vi "FL30XX - Copy.VI"() -> ()   [LabVIEW 2015]
uses:
  board.vis/Globals.vi
panel:
  out "String":string="with int trig:\nset exp.time accordingly\ncheck with scope!"
  in  "BlockSyncStart":string(combo)="S1"
  out "TDC 2":u16
  out "TDC 1":u16
  in  "startevent":bool
  in  "Scan Trig Input Sel":string(combo)="I"
  in  "rep time":dbl=20.0 format="%.3f"
  in  "FFT mode":string(combo)="Full Binning"
  in  "shutter open":bool
  in  "value black":u32
  in  "value white":u32=65535
  in  "show greyscale viewer":bool
  out "mean 3":dbl=42.0 format="%0#.1f"
  out "tRMS 3":dbl=42.0 format="%0#.1f"
  out "meanB":dbl format="%0#.1f"
  out "tRMSB":dbl format="%0#.1f"
  in  "Pixel for Graph":u32(slide)=660 max=3000 scale=0.0..1087.0
  in  "fast test\ncontinuous":bool
  out "One Pixel Graph":u16[][](graph)=[[65535, 65535, 7490, 7490, 7489, 7487, 7484, 7472, 7491, 7479]]
  in  "refresh":bool
  out "C 8":bool
  out "C 7":bool
  out "C 6":bool
  out "C 5":bool=TRUE
  out "C 4":bool=TRUE
  out "C 3":bool
  out "C 2":bool
  out "(LastCAM) \n        C1":bool
  out "cool_temp Reg":u32=411900038 format="%032b"
  in  "cool":u8 caption="(0 to 7)"
  in  "Offset":bool
  out "Signal Cam 4":u16[](graph)
  out "Signal Cam 3":u16[](graph)
  out "mean 2":dbl=42.0 format="%0#.1f"
  out "meanA":dbl=nan format="%0#.1f"
  in  "TRMS Pix":u32=1060
  out "tRMS 2":dbl=42.0 format="%0#.1f"
  in  "Board select":string(combo)
  in  "Initialize":bool
  in  "pattern hex (2)":u16=100 format="%x"
  out "pattern dec 2":fxp<+,14,14>=100.0
  in  "ADC mode 2":enum32{"1", "2", "3"}(radio)=enum."3"
  in  "camera gain":bool
  in  "About S0":bool
  in  "send all":bool
  in  "DAC 8/ 1":u16=53010
  in  "DAC 3/ 1":u16=53045
  in  "DAC 7/ 1":u16=53015
  in  "DAC 2/ 1":u16=53185
  in  "DAC 6/ 1":u16=53110
  in  "DAC 1/ 1":u16=53100
  in  "DAC 5/ 1":u16=53005
  in  "DAC 4/ 1":u16=53190
  in  "custom patt: 14bits pattern hex (14bit)":u16=100 format="%x"
  out "pattern dec":fxp<+,14,14>
  in  "ADC mode":enum32{"1", "2", "3"}(radio)=enum."3"
  out "Signal Cam 2":u16[](graph)
  in  "ext. trig. slope":enum32{"1", "2", "3"}(radio)
  out "tRMSA":dbl format="%0#.1f"
  in  "is FFT":bool=TRUE
  in  "Gain":bool
  in  "framewise\ncontinuous":bool
  out "curr_read_block":u8
  out "Measure ON":bool
  in  "no.of blocks (nob)":u32=1
  in  "block":u32(slide)=1 max=10 scale=0.9..1.0
  out "Signal Board 2 / Cam1":u16[](graph)=[486, 486, 486, 486, 0, 0, 0, 52, 0, 692, 692, 490, 486, 482, 487, 490, 495, 482, 495, 487, 492, 486, 500, 497, 493, 487, 497, 490, 490, 489, 487, 489, 486, 486, 495, 492, 489, 490, 498, 492, 493, 490, 500, 487, 492, 486, 504, 489, 487, 487, 490, 487, 495, 490, 493, 493, 490, 490, 490, 492, 492, 490, 487, 486, 487, 482, 495, 487, 490, 484, 489, 481, 490, 484, 489, 484, 486, 490, 484, 487, 497, 484, 481, 479, 484, 481, 481, 492, 490, 484, 490, 490, 490, 481, 484, 482, 484, 484, 482, 482, 492, 482, 479, 481, 489, 481, 495, 484, 497, 482, 486, 484, 487, 486, 484, 484, 486, 479, 482, 473, 492, 486, 481, 486, 493, 481, 487, 474, 486, 487, 490, 473, 489, 486, 482, 486, 486, 486, 486, 479, 460, 478, 470, 484, 470, 478, 481, 481, 467, 481, 473, 484, 471, 479, 481, 473, 473, 473, 468, 467, 463, 473, 463, 473, 468, 473, 471, 478, 473, 476, 473, 473, 470, 474, 478, 474, 471, 470, 470, 467, 470, 486, 478, 468, 463, 473, 471, 481, 476, 476, 471, 473, 463, 473, 468, 478, 459, 463, 471, 482, 478, 484, 465, 476, 468, 470, 474, 478, 468, 468, 476, 478, 470, 471, 462, 467, 462, 470, 473, 471, 467, 476, 465, 463, 465, 470, 459, 471, 465, 462, 470, 471, 470, 478, 465, 474, 470, 471, 465, 474, 459, 468, 465, 474, 467, 468, 468, 467, 468, 460, 465, 479, 463, 470, 463, 460, 471, 478, 460, 468, 463, 467, 468, 474, 457, 457, 457, 538, 531, 544, 533, 558, 534, 557, 536, 547, 533, 547, 549, 544, 534, 544, 534, 542, 544, 544, 538, 541, 538, 547, 538, 542, 536, 545, 547, 552, 544, 542, 544, 542, 544, 544, 549, 549, 553, 550, 542, 550, 538, 545, 544, 541, 539, 545, 544, 539, 550, 544, 541, 549, 527, 542, 539, 541, 539, 539, 541, 542, 541, 544, 534, 538, 533, 534, 538, 544, 547, 541, 539, 547, 538, 538, 542, 542, 527, 536, 536, 544, 533, 533, 536, 541, 536, 542, 528, 541, 527, 534, 528, 541, 539, 549, 544, 550, 536, 542, 541, 550, 541, 538, 533, 539, 536, 530, 534, 539, 534, 542, 541, 547, 533, 538, 527, 539, 538, 541, 530, 542, 533, 534, 538, 536, 538, 538, 538, 530, 522, 531, 533, 544, 536, 536, 525, 536, 538, 536, 538, 533, 530, 538, 534, 536, 525, 533, 525, 530, 528, 531, 528, 527, 522, 528, 530, 523, 530, 541, 523, 527, 530, 536, 528, 536, 525, 530, 533, 542, 527, 536, 538, 531, 531, 523, 525, 538, 523, 533, 527, 538, 527, 528, 520, 533, 520, 536, 531, 534, 530, 534, 525, 525, 525, 522, 523, 536, 534, 527, 525, 525, 531, 538, 527, 528, 520, 523, 533, 534, 516, 523, 517, 525, 523, 527, 523, 528, 525, 520, 525, 523, 525, 533, 527, 533, 528, 527, 523, 530, 520, 530, 520, 527, 520, 527, 517, 525, 522, 527, 525, 534, 523, 523, 522, 517, 528, 534, 517, 522, 527, 523, 516, 527, 522, 522, 522, 615, 613, 620, 613, 626, 615, 628, 617, 624, 605, 621, 618, 617, 609, 618, 621, 617, 612, 613, 605, 612, 610, 626, 612, 621, 607, 620, 613, 613, 623, 629, 617, 617, 613, 626, 617, 621, 610, 617, 609, 621, 617, 618, 618, 613, 612, 618, 626, 623, 623, 623, 612, 620, 615, 623, 610, 620, 607, 615, 609, 613, 613, 617, 607, 617, 612, 610, 609, 617, 613, 613, 609, 617, 609, 612, 612, 618, 607, 615, 610, 615, 609, 620, 612, 612, 610, 618, 610, 609, 601, 601, 607, 613, 605, 613, 615, 615, 612, 609, 612, 615, 609, 601, 607, 612, 604, 612, 596, 613, 612, 610, 612, 617, 609, 609, 612, 612, 615, 613, 607, 610, 607, 609, 613, 610, 609, 609, 609, 602, 593, 605, 607, 609, 593, 609, 607, 610, 609, 610, 604, 594, 602, 610, 602, 607, 594, 613, 594, 604, 604, 607, 602, 594, 601, 609, 602, 601, 602, 609, 598, 605, 602, 605, 604, 609, 601, 604, 607, 615, 599, 607, 610, 609, 607, 610, 607, 610, 612, 605, 602, 610, 596, 602, 594, 607, 602, 605, 599, 610, 601, 607, 590, 594, 601, 594, 594, 604, 602, 596, 602, 605, 599, 594, 588, 604, 593, 598, 596, 601, 591, 601, 594, 601, 601, 599, 587, 598, 593, 594, 594, 599, 601, 598, 599, 598, 602, 605, 593, 602, 598, 601, 596, 609, 598, 593, 588, 596, 601, 601, 593, 601, 594, 598, 601, 599, 599, 604, 591, 596, 593, 601, 601, 612, 596, 596, 596, 598, 593, 596, 594, 591, 593, 602, 598, 602, 596, 601, 594, 590, 583, 593, 598, 593, 588, 602, 594, 585, 587, 602, 591, 593, 593, 593, 591, 585, 599, 601, 591, 593, 599, 598, 594, 593, 587, 596, 590, 591, 591, 604, 598, 594, 596, 599, 590, 602, 601, 590, 582, 599, 583, 593, 580, 598, 591, 590, 587, 593, 588, 587, 585, 594, 590, 583, 590, 594, 585, 588, 583, 593, 593, 588, 585, 590, 588, 590, 596, 599, 588, 588, 590, 591, 591, 585, 587, 596, 583, 590, 585, 585, 579, 583, 582, 588, 587, 590, 588, 591, 579, 583, 588, 590, 582, 587, 580, 587, 585, 587, 587, 598, 590, 585, 582, 587, 593, 590, 585, 588, 588, 587, 591, 587, 596, 596, 596, 650, 651, 661, 662, 658, 651, 656, 654, 656, 654, 658, 656, 650, 651, 650, 654, 650, 658, 661, 653, 659, 654, 656, 658, 651, 653, 656, 658, 654, 658, 654, 654, 658, 654, 662, 653, 656, 653, 656, 656, 667, 653, 658, 654, 645, 648, 658, 659, 656, 658, 653, 650, 658, 650, 651, 653, 661, 643, 653, 654, 658, 651, 658, 640, 661, 645, 640, 646, 648, 653, 648, 650, 656, 648, 648, 658, 658, 642, 648, 661, 658, 646, 650, 653, 650, 645, 643, 645, 653, 643, 642, 646, 654, 648, 646, 651, 656, 648, 656, 642, 648, 640, 648, 646, 654, 654, 640, 645, 654, 645, 654, 651, 651, 650, 651, 645, 642, 650, 653, 653, 648, 651, 656, 651, 650, 646, 646, 646, 481, 482, 478, 486, 486, 486, 486, 486, 486, 486, 486, 486, 486, 486, 486, 486, 486, 486, 486, 486, 486, 486, 486, 486, 486, 486, 486, 486, 486, 486, 486, 486, 486, 486, 486, 486, 486, 486, 486, 486, 486, 486, 486, 486, 486, 486, 486, 486, 486, 486, 486, 486, 486]
  out "Signal Board 1 / Cam1":u16[](graph)=[6280, 6289, 0, 1, 0, 10, 0, 0, 0, 0, 6308, 6311, 6305, 7303, 7306, 7305, 7298, 7309, 7318, 7312, 7317, 7306, 7300, 7301, 7287, 7279, 7286, 7287, 7288, 7284, 7286, 7285, 7270, 7282, 7282, 7261, 7269, 7267, 7263, 7261, 7274, 7261, 7263, 7266, 7264, 7271, 7253, 7245, 7254, 7250, 7257, 7250, 7235, 7242, 7238, 7242, 7236, 7239, 7237, 7237, 7237, 7238, 7231, 7224, 7231, 7221, 7222, 7224, 7210, 7213, 7215, 7217, 7219, 7225, 7215, 7211, 7219, 7221, 7209, 7207, 7208, 7206, 7194, 7206, 7213, 7200, 7196, 7193, 7205, 7190, 7191, 7203, 7205, 7199, 7187, 7196, 7198, 7179, 7188, 7191, 7186, 7185, 7189, 7184, 7181, 7177, 7192, 7182, 7181, 7173, 7180, 7174, 7171, 7173, 7169, 7174, 7166, 7161, 7138, 7168, 7165, 7168, 7167, 7171, 7157, 7169, 7155, 7156, 7173, 7153, 7166, 7156, 7153, 7150, 7155, 7150, 7153, 7142, 7138, 7135, 7140, 7156, 7152, 7147, 7145, 7142, 7147, 7135, 7133, 7146, 7135, 7152, 7134, 7129, 7141, 7137, 7140, 7130, 7139, 7144, 7129, 7142, 7133, 7131, 7121, 7130, 7125, 7135, 7139, 7126, 7131, 7134, 7138, 7127, 7120, 7137, 7121, 7133, 7144, 7136, 7135, 7133, 7138, 7134, 7135, 7141, 7145, 7149, 7150, 7144, 7143, 7157, 7165, 7156, 7152, 7146, 7152, 7150, 7155, 7159, 7150, 7160, 7145, 7139, 7147, 7154, 7134, 7153, 7144, 7138, 7141, 7146, 7148, 7134, 7148, 7140, 7153, 7138, 7143, 7134, 7155, 7157, 7153, 7147, 7149, 7150, 7151, 7141, 7135, 7142, 7136, 7146, 7143, 7152, 7147, 7139, 7144, 7152, 7150, 7129, 7136, 7137, 7149, 7145, 7132, 7144, 7138, 7141, 7145, 7142, 7141, 7145, 7142, 7140, 7143, 7138, 7145, 7154, 7139, 7148, 7149, 7150, 7135, 7149, 7145, 7151, 7151, 7147, 7143, 7148, 7145, 7142, 7144, 7149, 7158, 7148, 7149, 7148, 7151, 7154, 7148, 7139, 7144, 7142, 7145, 7142, 7150, 7154, 7138, 7142, 7152, 7145, 7146, 7147, 7146, 7140, 7144, 7146, 7148, 7152, 7152, 7159, 7154, 7146, 7155, 7157, 7147, 7153, 7146, 7156, 7155, 7153, 7148, 7153, 7154, 7159, 7155, 7154, 7157, 7152, 7157, 7155, 7147, 7154, 7154, 7151, 7154, 7168, 7167, 7164, 7168, 7161, 7165, 7168, 7147, 7156, 7157, 7162, 7160, 7160, 7164, 7169, 7163, 7168, 7170, 7161, 7174, 7162, 7159, 7166, 7167, 7162, 7169, 7168, 7158, 7162, 7163, 7174, 7160, 7158, 7167, 7168, 7176, 7178, 7162, 7176, 7176, 7158, 7178, 7166, 7174, 7162, 7168, 7186, 7170, 7171, 7163, 7176, 7158, 7177, 7178, 7169, 7166, 7168, 7165, 7179, 7174, 7177, 7180, 7186, 7190, 7181, 7180, 7181, 7169, 7179, 7174, 7178, 7196, 7183, 7189, 7193, 7187, 7194, 7184, 7185, 7184, 7196, 7198, 7193, 7202, 7198, 7203, 7197, 7187, 7200, 7197, 7197, 7205, 7201, 7206, 7212, 7186, 7199, 7206, 7196, 7212, 7213, 7217, 7209, 7221, 7204, 7212, 7209, 7218, 7220, 7215, 7222, 7228, 7218, 7223, 7218, 7231, 7219, 7227, 7219, 7223, 7228, 7231, 7224, 7234, 7236, 7240, 7227, 7237, 7243, 7241, 7240, 7228, 7238, 7233, 7241, 7233, 7238, 7244, 7240, 7240, 7232, 7252, 7238, 7247, 7249, 7249, 7247, 7248, 7259, 7250, 7256, 7256, 7263, 7258, 7259, 7261, 7266, 7274, 7271, 7262, 7261, 7258, 7259, 7266, 7269, 7274, 7271, 7280, 7282, 7271, 7290, 7275, 7288, 7288, 7287, 7286, 7275, 7297, 7289, 7286, 7289, 7297, 7284, 7307, 7299, 7295, 7293, 7311, 7298, 7297, 7305, 7310, 7298, 7306, 7306, 7320, 7310, 7313, 7320, 7313, 7312, 7313, 7313, 7325, 7321, 7325, 7309, 7328, 7335, 7326, 7321, 7339, 7324, 7332, 7333, 7333, 7334, 7343, 7331, 7364, 7337, 7328, 7338, 7348, 7355, 7341, 7350, 7368, 7369, 7362, 7361, 7369, 7368, 7357, 7377, 7362, 7365, 7364, 7371, 7363, 7371, 7384, 7374, 7385, 7370, 7370, 7387, 7394, 7380, 7383, 7398, 7395, 7393, 7389, 7402, 7402, 7394, 7387, 7406, 7388, 7403, 7403, 7404, 7404, 7413, 7401, 7407, 7410, 7406, 7405, 7402, 7408, 7409, 7415, 7420, 7416, 7416, 7419, 7422, 7408, 7426, 7424, 7428, 7431, 7420, 7433, 7430, 7421, 7427, 7438, 7431, 7440, 7433, 7440, 7442, 7446, 7441, 7453, 7443, 7441, 7450, 7447, 7459, 7441, 7457, 7461, 7447, 7448, 7461, 7455, 7467, 7465, 7450, 7466, 7463, 7464, 7463, 7461, 7466, 7465, 7478, 7479, 7466, 7471, 7482, 7497, 7463, 7484, 7490, 7495, 7474, 7488, 7489, 7479, 7498, 7493, 7489, 7490, 7498, 7487, 7487, 7495, 7501, 7491, 7491, 7509, 7496, 7507, 7506, 7495, 7500, 7505, 7505, 7500, 7511, 7513, 7504, 7504, 7509, 7520, 7526, 7518, 7517, 7521, 7519, 7514, 7534, 7523, 7518, 7521, 7529, 7536, 7530, 7534, 7532, 7510, 7521, 7529, 7530, 7534, 7522, 7545, 7530, 7531, 7539, 7540, 7553, 7545, 7542, 7531, 7542, 7540, 7552, 7565, 7548, 7554, 7551, 7554, 7548, 7564, 7574, 7565, 7555, 7560, 7572, 7561, 7563, 7571, 7556, 7569, 7571, 7568, 7569, 7585, 7572, 7577, 7574, 7568, 7591, 7583, 7579, 7580, 7590, 7586, 7592, 7604, 7604, 7597, 7593, 7600, 7606, 7620, 7616, 7618, 7602, 7616, 7621, 7609, 7633, 7618, 7629, 7640, 7638, 7630, 7634, 7630, 7631, 7642, 7639, 7627, 7635, 7646, 7656, 7663, 7653, 7654, 7645, 7655, 7656, 7653, 7665, 7659, 7654, 7671, 7661, 7672, 7683, 7675, 7677, 7666, 7669, 7654, 7678, 7676, 7674, 7678, 7679, 7674, 7672, 7677, 7693, 7688, 7685, 7681, 7691, 7693, 7702, 7691, 7691, 7698, 7694, 7696, 7698, 7682, 7694, 7698, 7689, 7699, 7699, 7682, 7700, 7689, 7696, 7705, 7686, 7702, 7693, 7686, 7689, 7687, 7685, 7694, 7705, 7689, 7694, 7692, 7680, 7706, 7694, 7690, 7691, 7683, 7686, 7676, 7662, 7664, 7676, 7655, 7674, 7650, 7660, 7644, 7643, 7642, 7635, 7625, 7632, 7621, 7605, 7603, 7597, 7598, 7582, 7575, 7568, 7568, 7568, 7565, 7554, 7533, 7529, 7532, 7507, 7510, 7508, 7509, 7491, 7470, 7468, 7464, 7465, 7445, 7433, 7425, 7409, 7410, 7398, 7399, 7379, 7373, 7365, 7346, 7341, 7322, 7325, 7308, 7296, 7289, 7281, 7271, 7251, 7253, 7243, 7223, 7201, 7189, 7167, 7174, 7161, 7135, 7122, 7095, 7082, 7070, 7055, 7045, 7017, 6997, 6995, 6973, 6966, 6960, 6928, 6942, 6926, 6922, 6915, 6901, 6896, 6883, 6873, 6879, 6874, 6860, 6851, 6855, 6841, 6833, 6827, 6822, 6813, 6811, 6800, 6810, 6803, 6788, 6782, 6786, 6772, 6767, 6771, 6765, 6752, 6758, 6753, 6743, 6737, 6745, 6733, 6725, 6717, 6728, 6717, 6720, 6711, 6708, 6706, 6702, 6705, 6695, 6687, 6687, 6689, 6676, 6676, 6679, 6665, 6663, 6640, 6654, 6656, 6650, 6644, 6645, 6644, 6639, 6631, 6634, 6631, 6620, 6626, 6621, 6620, 6611, 6612, 6609, 6615, 6607, 6605, 6596, 6604, 6596, 6589, 6586, 6585, 6589, 6583, 6582, 6576, 6578, 6563, 6579, 6574, 6565, 6565, 6562, 6560, 6559, 6551, 6547, 6556, 6546, 6549, 6535, 6533, 6539, 6541, 6540, 6527, 6525, 6528, 6523, 6525, 6524, 6520, 6522, 6519, 6518, 6505, 6510, 6503, 6502, 6286, 6279, 6278, 6281, 6279, 6279, 6286, 6279, 6280, 6282, 6285, 6282, 6284, 6285, 6282, 6280, 6285, 6281, 6283, 6283, 6280, 6276, 6282, 6282, 6283, 6276, 6281, 6277, 6282, 6277, 6279, 6277, 6281, 0, 0, 65535, 65535, 6279, 6283]
  out "# boards \ndetected":u8=1
  in  "alloc mem":bool
  out "FREE \nRAM MB":dbl=29529.31640625
  out "BUILT-IN\nRAM MB":dbl=32640.29296875
  out "SEC":dbl=0.005
  out "MB RAM":dbl=0.0103759765625
  in  "DAT in 10ns":u32
  in  "stop all":bool
  in  "start":bool
  in  "sample":u32(slide)=10 max=3000 scale=0.9..4.0
  in  "no.of samples (nos)":u32=4
  in  "exposuretime[ms]":dbl=1.0 format="%.3f"
  # "Put the right values in this frame\n           and press \"Initialize\""
  # "press Esc to\nstop measurement"
  # "exit here"
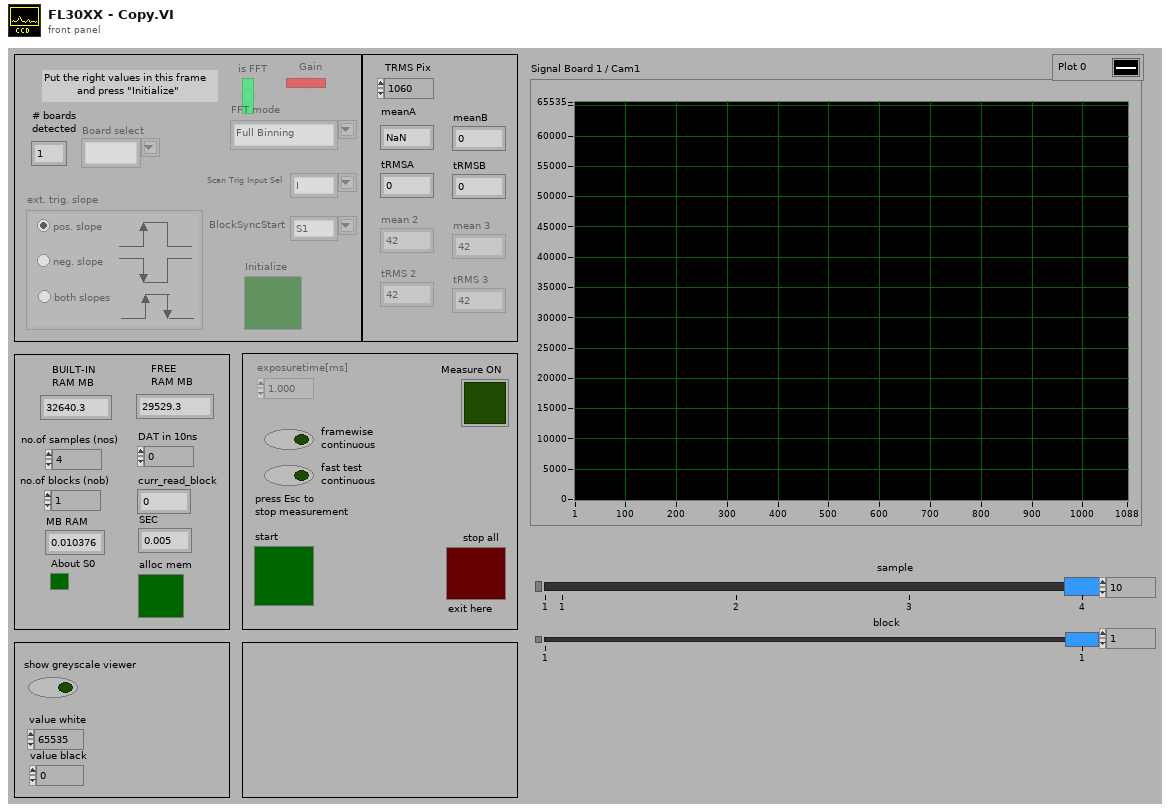
[diagram p1: front panel]
types:
  T1 = enum8{"Enabled", "Disabled", "Disabled and Grayed Out"}
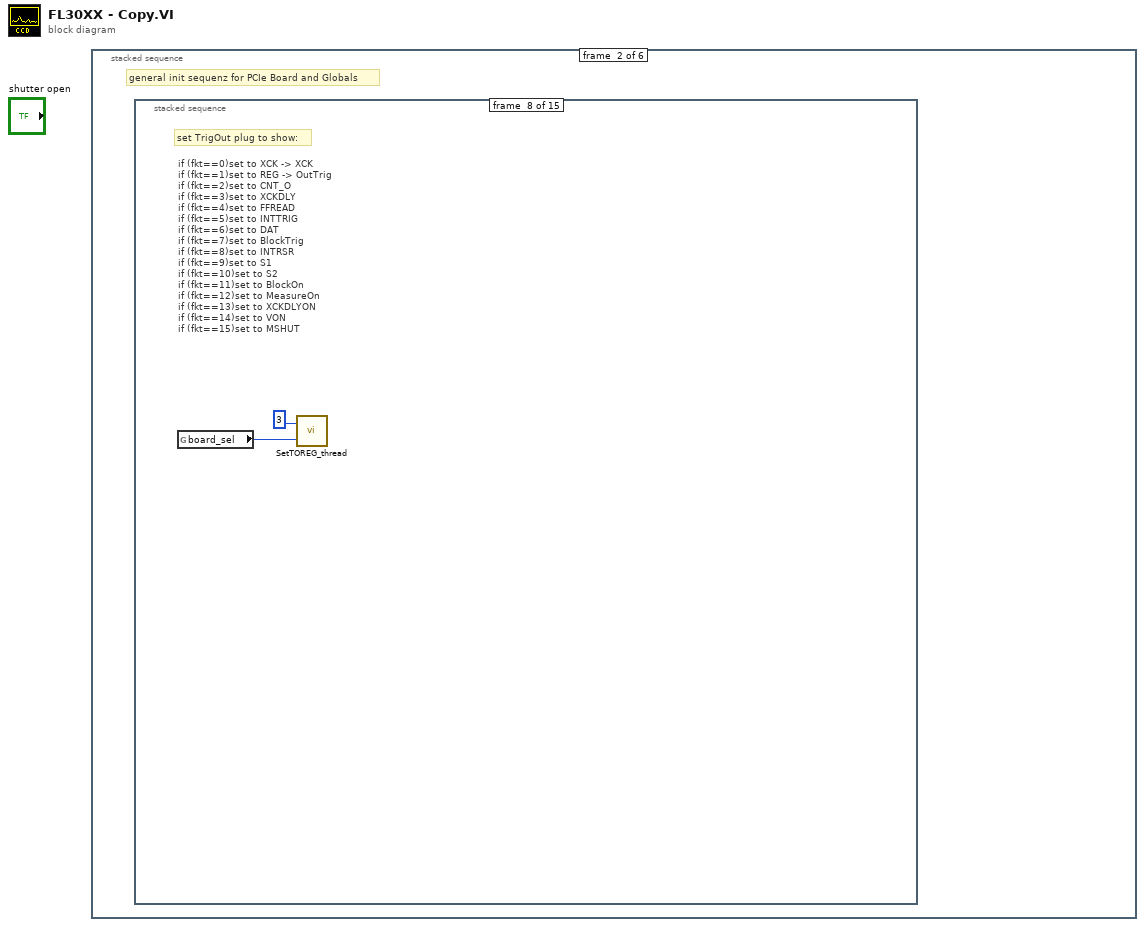
[diagram p0: block diagram]
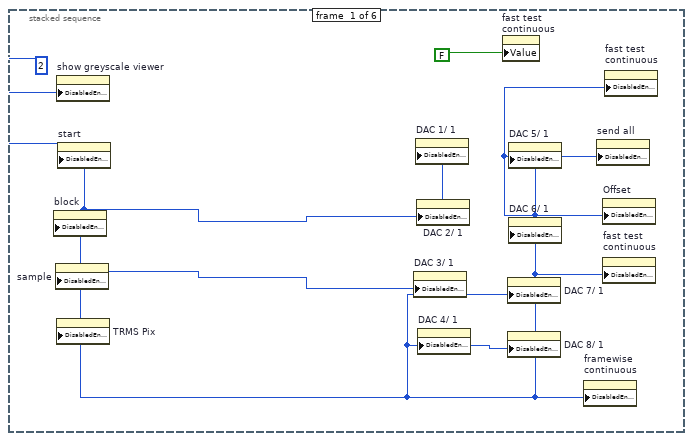
[diagram p2: hidden frame]
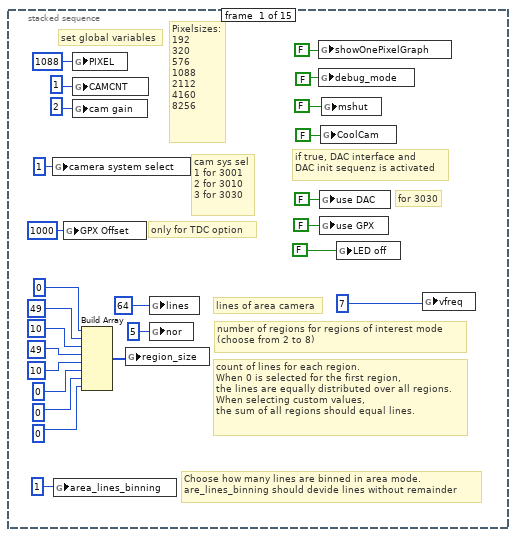
[diagram p3: hidden frame]
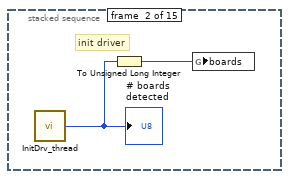
[diagram p4: hidden frame]
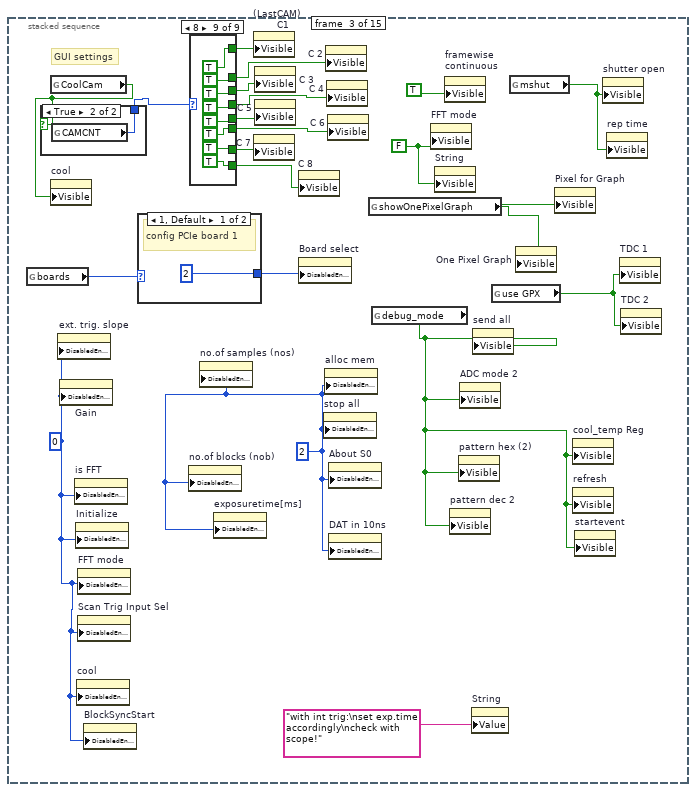
[diagram p5: hidden frame]
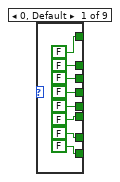
[diagram p6: hidden frame]
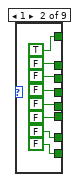
[diagram p7: hidden frame]
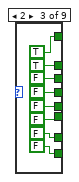
[diagram p8: hidden frame]
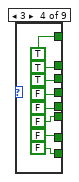
[diagram p9: hidden frame]
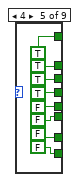
[diagram p10: hidden frame]
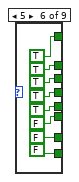
[diagram p11: hidden frame]
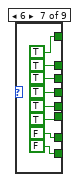
[diagram p12: hidden frame]
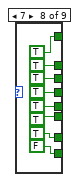
[diagram p13: hidden frame]
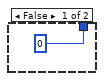
[diagram p14: hidden frame]
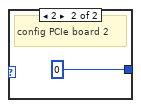
[diagram p15: hidden frame]
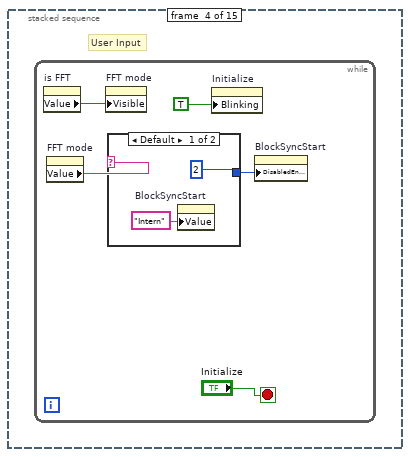
[diagram p16: hidden frame]
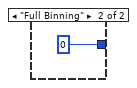
[diagram p17: hidden frame]
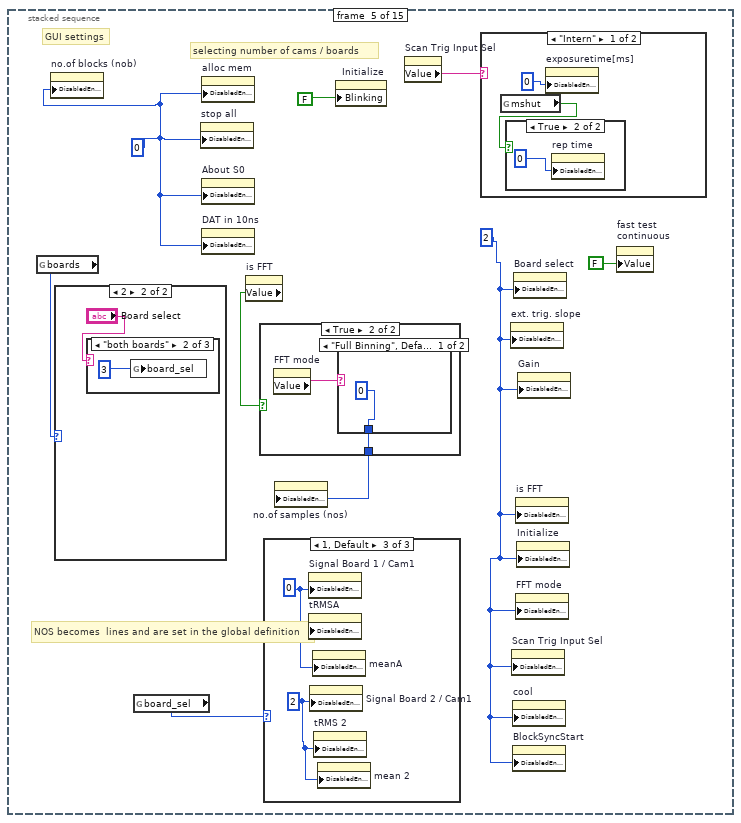
[diagram p18: hidden frame]
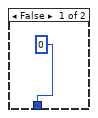
[diagram p19: hidden frame]
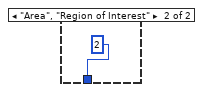
[diagram p20: hidden frame]
diagram:
  n1 = stacked-sequence {
    frame #0 {
      w1 = 2
      n2 = property on="block" class="Slide (strict)"("DisabledEnum"=w1) -> ()  [unwired: 2 in, 2 out]
      n3 = property on="sample" class="Slide (strict)"("DisabledEnum"=w1) -> ()  [unwired: 2 in, 2 out]
      n4 = property on="show greyscale viewer" class="Bool (strict)"("DisabledEnum"=w1) -> ()  [unwired: 2 in, 2 out]
      n5 = property on="TRMS Pix" class="DigNum (strict)"("DisabledEnum"=w1) -> ()  [unwired: 2 in, 2 out]
      n6 = property on="start" class="Bool (strict)"("DisabledEnum"=w1) -> ()  [unwired: 2 in, 2 out]
      n7 = property on="DAC 3/ 1" class="DigNum (strict)"("DisabledEnum"=w1) -> ()  [unwired: 2 in, 2 out]
      n8 = property on="DAC 1/ 1" class="DigNum (strict)"("DisabledEnum"=w1) -> ()  [unwired: 2 in, 2 out]
      n9 = property on="DAC 2/ 1" class="DigNum (strict)"("DisabledEnum"=w1) -> ()  [unwired: 2 in, 2 out]
      n10 = property on="DAC 4/ 1" class="DigNum (strict)"("DisabledEnum"=w1) -> ()  [unwired: 2 in, 2 out]
      n11 = property on="fast test\ncontinuous" class="Bool (strict)"("Value"=FALSE) -> ()  [unwired: 2 in, 2 out]
      n12 = property on="DAC 7/ 1" class="DigNum (strict)"("DisabledEnum"=w1) -> ()  [unwired: 2 in, 2 out]
      n13 = property on="DAC 8/ 1" class="DigNum (strict)"("DisabledEnum"=w1) -> ()  [unwired: 2 in, 2 out]
      n14 = property on="DAC 5/ 1" class="DigNum (strict)"("DisabledEnum"=w1) -> ()  [unwired: 2 in, 2 out]
      n15 = property on="DAC 6/ 1" class="DigNum (strict)"("DisabledEnum"=w1) -> ()  [unwired: 2 in, 2 out]
      n16 = property on="framewise\ncontinuous" class="Bool (strict)"("DisabledEnum"=w1) -> ()  [unwired: 2 in, 2 out]
      n17 = property on="send all" class="Bool (strict)"("DisabledEnum"=w1) -> ()  [unwired: 2 in, 2 out]
      n18 = property on="Offset" class="Bool (strict)"("DisabledEnum"=w1) -> ()  [unwired: 2 in, 2 out]
      n19 = property on="fast test\ncontinuous" class="Bool (strict)"("DisabledEnum"=w1) -> ()  [unwired: 2 in, 2 out]
      n20 = property on="fast test\ncontinuous" class="Bool (strict)"("DisabledEnum"=w1) -> ()  [unwired: 2 in, 2 out]
    }
    frame #1 {
      # "general init sequenz for PCIe Board and Globals"
      n21 = stacked-sequence {
        frame #0 {
          # "Choose how many lines are binned in area mode.\nare_lines_binning should devide lines without remainder"
          # "count of lines for each region.\nWhen 0 is selected for the first region,\nthe lines are equally distributed over all regions.\nWhen selecting custom values,\nthe sum of all regions should equal lines."
          # "number of regions for regions of interest mode\n(choose from 2 to 8)"
          # "lines of area camera"
          # "only for TDC option"
          # "Pixelsizes:\n192\n320\n576\n1088\n2112\n4160\n8256"
          # "if true, DAC interface and \nDAC init sequenz is activated"
          # "for 3030"
          # "set global variables"
          # "cam sys sel\n1 for 3001\n2 for 3010\n3 for 3030"
          n22 = global write "Globals.vi" "camera system select"(u8 1) -> ()
          n23 = global write "Globals.vi" "area_lines_binning"(u32 1) -> ()
          n24 = global write "Globals.vi" "GPX Offset"(u32 1000) -> ()
          n25 = global write "Globals.vi" "PIXEL"(u32 1088) -> ()
          n26 = global write "Globals.vi" "CAMCNT"(u32 1) -> ()
          n27 = global write "Globals.vi" "cam gain"(u32 2) -> ()
          n28 = Build Array(u8 0, u8 49, u8 10, u8 49, u8 10, u8 0, u8 0, u8 0) -> (w6:u8[])
          n29 = global write "Globals.vi" "region_size"(w6) -> ()
          n30 = global write "Globals.vi" "lines"(u32 64) -> ()
          n31 = global write "Globals.vi" "nor"(u32 5) -> ()
          n32 = global write "Globals.vi" "showOnePixelGraph"(FALSE) -> ()
          n33 = global write "Globals.vi" "debug_mode"(FALSE) -> ()
          n34 = global write "Globals.vi" "use DAC"(FALSE) -> ()
          n35 = global write "Globals.vi" "use GPX"(FALSE) -> ()
          n36 = global write "Globals.vi" "CoolCam"(FALSE) -> ()
          n37 = global write "Globals.vi" "mshut"(FALSE) -> ()
          n38 = global write "Globals.vi" "LED off"(FALSE) -> ()
          n39 = global write "Globals.vi" "vfreq"(u8 7) -> ()
        }
        frame #1 {
          # "init driver"
          n40 = call "InitDrv_thread.vi"() -> ("Boards"=w28:u8)  [unwired: 1 in]
          "# boards \ndetected" <- w28
          n41 = To Unsigned Long Integer(number=w28) -> (unsigned 32bit integer=w29:u32)
          n42 = global write "Globals.vi" "boards"(w29) -> ()
        }
        frame #2 {
          w32 = FALSE
          w30 = 0
          w33 = 2
          # "GUI settings"
          n43 = global read "Globals.vi" "boards"() -> (w49:u32)
          n44 = global read "Globals.vi" "CoolCam"() -> (w38:bool)
          n45 = case shown="True" w38 {
            tunnel: [u32 0 w124] -> w47
            frame False {
            }
            frame True {
              n46 = global read "Globals.vi" "CAMCNT"() -> (w124:u32)
            }
          }
          n47 = property on="cool" class="DigNum (strict)"("Visible"=w38) -> ()  [unwired: 2 in, 2 out]
          n48 = property on="ext. trig. slope" class="RadioBtnsControl (strict)"("DisabledEnum"=w30) -> ()  [unwired: 2 in, 2 out]
          n49 = property on="Gain" class="Bool (strict)"("DisabledEnum"=w30) -> ()  [unwired: 2 in, 2 out]
          n50 = property on="is FFT" class="Bool (strict)"("DisabledEnum"=w30) -> ()  [unwired: 2 in, 2 out]
          n51 = property on="Initialize" class="Bool (strict)"("DisabledEnum"=w30) -> ()  [unwired: 2 in, 2 out]
          n52 = property on="cool" class="DigNum (strict)"("DisabledEnum"=w30) -> ()  [unwired: 2 in, 2 out]
          n53 = property on="FFT mode" class="CmbBox"("DisabledEnum"=w30) -> ()  [unwired: 2 in, 2 out]
          n54 = property on="Scan Trig Input Sel" class="CmbBox"("DisabledEnum"=w30) -> ()  [unwired: 2 in, 2 out]
          n55 = property on="BlockSyncStart" class="CmbBox"("DisabledEnum"=w30) -> ()  [unwired: 2 in, 2 out]
          n56 = case shown="1, Default" w49 {
            tunnel: [2 0] -> w50
            frame 1, Default {
              # "config PCIe board 1"
            }
            frame 2 {
              # "config PCIe board 2"
            }
          }
          n57 = property on="no.of blocks (nob)" class="DigNum (strict)"("DisabledEnum"=w33) -> ()  [unwired: 2 in, 2 out]
          n58 = case shown="8" w47 {
            tunnel: [FALSE TRUE TRUE TRUE TRUE TRUE TRUE TRUE TRUE] -> w46
            tunnel: [FALSE FALSE FALSE TRUE TRUE TRUE TRUE TRUE TRUE] -> w45
            tunnel: [FALSE FALSE FALSE FALSE TRUE TRUE TRUE TRUE TRUE] -> w44
            tunnel: [FALSE FALSE FALSE FALSE FALSE TRUE TRUE TRUE TRUE] -> w43
            tunnel: [FALSE FALSE FALSE FALSE FALSE FALSE TRUE TRUE TRUE] -> w42
            tunnel: [FALSE FALSE FALSE FALSE FALSE FALSE FALSE TRUE TRUE] -> w41
            tunnel: [FALSE FALSE FALSE FALSE FALSE FALSE FALSE FALSE TRUE] -> w40
            tunnel: [FALSE FALSE TRUE TRUE TRUE TRUE TRUE TRUE TRUE] -> w39
            frame 0, Default {
            }
            frame 1 {
            }
            frame 2 {
            }
            frame 3 {
            }
            frame 4 {
            }
            frame 5 {
            }
            frame 6 {
            }
            frame 7 {
            }
            frame 8 {
            }
          }
          n59 = property on="no.of samples (nos)" class="DigNum (strict)"("DisabledEnum"=w33) -> ()  [unwired: 2 in, 2 out]
          n60 = property on="exposuretime[ms]" class="DigNum (strict)"("DisabledEnum"=w33) -> ()  [unwired: 2 in, 2 out]
          n61 = property on="(LastCAM) \n        C1" class="Bool (strict)"("Visible"=w46) -> ()  [unwired: 2 in, 2 out]
          n62 = property on="C 7" class="Bool (strict)"("Visible"=w41) -> ()  [unwired: 2 in, 2 out]
          n63 = property on="C 3" class="Bool (strict)"("Visible"=w45) -> ()  [unwired: 2 in, 2 out]
          n64 = property on="C 5" class="Bool (strict)"("Visible"=w43) -> ()  [unwired: 2 in, 2 out]
          n65 = property on="C 8" class="Bool (strict)"("Visible"=w40) -> ()  [unwired: 2 in, 2 out]
          n66 = property on="Board select" class="CmbBox"("DisabledEnum"=w50) -> ()  [unwired: 2 in, 2 out]
          n67 = property on="stop all" class="Bool (strict)"("DisabledEnum"=w33) -> ()  [unwired: 2 in, 2 out]
          n68 = property on="alloc mem" class="Bool (strict)"("DisabledEnum"=w33) -> ()  [unwired: 2 in, 2 out]
          n69 = property on="C 2" class="Bool (strict)"("Visible"=w39) -> ()  [unwired: 2 in, 2 out]
          n70 = property on="C 4" class="Bool (strict)"("Visible"=w44) -> ()  [unwired: 2 in, 2 out]
          n71 = property on="C 6" class="Bool (strict)"("Visible"=w42) -> ()  [unwired: 2 in, 2 out]
          n72 = property on="About S0" class="Bool (strict)"("DisabledEnum"=w33) -> ()  [unwired: 2 in, 2 out]
          n73 = property on="DAT in 10ns" class="DigNum (strict)"("DisabledEnum"=w33) -> ()  [unwired: 2 in, 2 out]
          n74 = global read "Globals.vi" "showOnePixelGraph"() -> (w37:bool)
          n75 = global read "Globals.vi" "debug_mode"() -> (w35:bool)
          n76 = property on="FFT mode" class="CmbBox"("Visible"=w32) -> ()  [unwired: 2 in, 2 out]
          n77 = property on="String" class="Str"("Visible"=w32) -> ()  [unwired: 2 in, 2 out]
          n78 = property on="framewise\ncontinuous" class="Bool (strict)"("Visible"=TRUE) -> ()  [unwired: 2 in, 2 out]
          n79 = property on="pattern dec 2" class="DigNum (strict)"("Visible"=w35) -> ()  [unwired: 2 in, 2 out]
          n80 = property on="pattern hex (2)" class="DigNum (strict)"("Visible"=w35) -> ()  [unwired: 2 in, 2 out]
          n81 = property on="ADC mode 2" class="RadioBtnsControl (strict)"("Visible"=w35) -> ()  [unwired: 2 in, 2 out]
          n82 = property on="String" class="Str"("Value"="with int trig:\nset exp.time accordingly\ncheck with scope!") -> ()  [unwired: 2 in, 2 out]
          n83 = property on="send all" class="Bool (strict)"("Visible"=w35) -> ()  [unwired: 2 in, 2 out]
          n84 = global read "Globals.vi" "use GPX"() -> (w34:bool)
          n85 = global read "Globals.vi" "mshut"() -> (w36:bool)
          n86 = property on="One Pixel Graph" class="WFGraph (strict)"("Visible"=w37) -> ()  [unwired: 2 in, 2 out]
          n87 = property on="Pixel for Graph" class="Slide (strict)"("Visible"=w37) -> ()  [unwired: 2 in, 2 out]
          n88 = property on="cool_temp Reg" class="DigNum (strict)"("Visible"=w35) -> ()  [unwired: 2 in, 2 out]
          n89 = property on="refresh" class="Bool (strict)"("Visible"=w35) -> ()  [unwired: 2 in, 2 out]
          n90 = property on="startevent" class="Bool (strict)"("Visible"=w35) -> ()  [unwired: 2 in, 2 out]
          n91 = property on="shutter open" class="Bool (strict)"("Visible"=w36) -> ()  [unwired: 2 in, 2 out]
          n92 = property on="rep time" class="DigNum (strict)"("Visible"=w36) -> ()  [unwired: 2 in, 2 out]
          n93 = property on="TDC 1" class="DigNum (strict)"("Visible"=w34) -> ()  [unwired: 2 in, 2 out]
          n94 = property on="TDC 2" class="DigNum (strict)"("Visible"=w34) -> ()  [unwired: 2 in, 2 out]
        }
        frame #3 {
          # "User Input"
          n95 = while {
            stop <- "Initialize" stop-if-true
            n96 = property on="is FFT" class="Bool (strict)"() -> ("Value"=w129:bool)  [unwired: 2 in, 2 out]
            n97 = property on="FFT mode" class="CmbBox"() -> ("Value"=w128:string)  [unwired: 2 in, 2 out]
            n98 = property on="FFT mode" class="CmbBox"("Visible"=w129) -> ()  [unwired: 2 in, 2 out]
            n99 = case shown="Default" w128 {
              tunnel: [2 0] -> w127
              frame Default {
                n100 = property on="BlockSyncStart" class="CmbBox"("Value"="Intern") -> ()  [unwired: 2 in, 2 out]
              }
              frame "Full Binning" {
              }
            }
            n101 = property on="Initialize" class="Bool (strict)"("Blinking"=TRUE) -> ()  [unwired: 2 in, 2 out]
            n102 = property on="BlockSyncStart" class="CmbBox"("DisabledEnum"=w127) -> ()  [unwired: 2 in, 2 out]
          }
        }
        frame #4 {
          w136 = u8 2
          w143 = i8 0
          # "NOS becomes  lines and are set in the global definition"
          # "GUI settings"
          # "selecting number of cams / boards"
          n103 = global read "Globals.vi" "boards"() -> (w141:u32)
          n104 = property on="no.of blocks (nob)" class="DigNum (strict)"("DisabledEnum"=w143) -> ()  [unwired: 2 in, 2 out]
          n105 = case shown="2" w141 {
            frame 1, Default {
              n106 = global write "Globals.vi" "board_sel"(u32 1) -> ()
            }
            frame 2 {
              n107 = case shown="\"both boards\"" "Board select" {
                frame "board 2" {
                  n108 = global write "Globals.vi" "board_sel"(u32 2) -> ()
                }
                frame "both boards" {
                  n109 = global write "Globals.vi" "board_sel"(u32 3) -> ()
                }
                frame "board 1", Default {
                  n110 = global write "Globals.vi" "board_sel"(u32 1) -> ()
                }
              }
            }
          }
          n111 = global read "Globals.vi" "board_sel"() -> (w140:u32)
          n112 = property on="stop all" class="Bool (strict)"("DisabledEnum"=w143) -> ()  [unwired: 2 in, 2 out]
          n113 = property on="alloc mem" class="Bool (strict)"("DisabledEnum"=w143) -> ()  [unwired: 2 in, 2 out]
          n114 = property on="About S0" class="Bool (strict)"("DisabledEnum"=w143) -> ()  [unwired: 2 in, 2 out]
          n115 = property on="DAT in 10ns" class="DigNum (strict)"("DisabledEnum"=w143) -> ()  [unwired: 2 in, 2 out]
          n116 = property on="is FFT" class="Bool (strict)"() -> ("Value"=w137:bool)  [unwired: 2 in, 2 out]
          n117 = case shown="True" w137 {
            tunnel: [u8 0 w145] -> w138
            frame False {
            }
            frame True {
              n118 = property on="FFT mode" class="CmbBox"() -> ("Value"=w146:string)  [unwired: 2 in, 2 out]
              n119 = case shown="\"Full Binning\", Default" w146 {
                tunnel: [i8 0 i8 2] -> w145
                frame "Full Binning", Default {
                }
                frame "Area", "Region of Interest" {
                }
              }
            }
          }
          n120 = case shown="1, Default" w140 {
            frame 2 {
              w157 = 0
              w158 = 2
              n121 = property on="Signal Board 1 / Cam1" class="WFGraph (strict)"("DisabledEnum"=w158) -> ()  [unwired: 2 in, 2 out]
              n122 = property on="tRMSA" class="DigNum (strict)"("DisabledEnum"=w158) -> ()  [unwired: 2 in, 2 out]
              n123 = property on="Signal Board 2 / Cam1" class="WFGraph (strict)"("DisabledEnum"=w157) -> ()  [unwired: 2 in, 2 out]
              n124 = property on="meanA" class="DigNum (strict)"("DisabledEnum"=w158) -> ()  [unwired: 2 in, 2 out]
              n125 = property on="tRMS 2" class="DigNum (strict)"("DisabledEnum"=w157) -> ()  [unwired: 2 in, 2 out]
              n126 = property on="mean 2" class="DigNum (strict)"("DisabledEnum"=w157) -> ()  [unwired: 2 in, 2 out]
            }
            frame 3 {
              w159 = 0
              w160 = 0
              n127 = property on="Signal Board 1 / Cam1" class="WFGraph (strict)"("DisabledEnum"=w160) -> ()  [unwired: 2 in, 2 out]
              n128 = property on="tRMSA" class="DigNum (strict)"("DisabledEnum"=w160) -> ()  [unwired: 2 in, 2 out]
              n129 = property on="Signal Board 2 / Cam1" class="WFGraph (strict)"("DisabledEnum"=w159) -> ()  [unwired: 2 in, 2 out]
              n130 = property on="meanA" class="DigNum (strict)"("DisabledEnum"=w160) -> ()  [unwired: 2 in, 2 out]
              n131 = property on="tRMS 2" class="DigNum (strict)"("DisabledEnum"=w159) -> ()  [unwired: 2 in, 2 out]
              n132 = property on="mean 2" class="DigNum (strict)"("DisabledEnum"=w159) -> ()  [unwired: 2 in, 2 out]
            }
            frame 1, Default {
              w161 = 2
              w162 = 0
              n133 = property on="Signal Board 1 / Cam1" class="WFGraph (strict)"("DisabledEnum"=w162) -> ()  [unwired: 2 in, 2 out]
              n134 = property on="tRMSA" class="DigNum (strict)"("DisabledEnum"=w162) -> ()  [unwired: 2 in, 2 out]
              n135 = property on="Signal Board 2 / Cam1" class="WFGraph (strict)"("DisabledEnum"=w161) -> ()  [unwired: 2 in, 2 out]
              n136 = property on="meanA" class="DigNum (strict)"("DisabledEnum"=w162) -> ()  [unwired: 2 in, 2 out]
              n137 = property on="tRMS 2" class="DigNum (strict)"("DisabledEnum"=w161) -> ()  [unwired: 2 in, 2 out]
              n138 = property on="mean 2" class="DigNum (strict)"("DisabledEnum"=w161) -> ()  [unwired: 2 in, 2 out]
            }
          }
          n139 = property on="no.of samples (nos)" class="DigNum (strict)"("DisabledEnum"=w138) -> ()  [unwired: 2 in, 2 out]
          n140 = property on="Initialize" class="Bool (strict)"("Blinking"=FALSE) -> ()  [unwired: 2 in, 2 out]
          n141 = property on="Scan Trig Input Sel" class="CmbBox"() -> ("Value"=w135:string)  [unwired: 2 in, 2 out]
          n142 = case shown="\"Intern\"" w135 {
            frame "Intern" {
              n143 = global read "Globals.vi" "mshut"() -> (w149:bool)
              n144 = case shown="True" w149 {
                frame False {
                  n145 = property on="rep time" class="DigNum (strict)"("DisabledEnum"=i8 2) -> ()  [unwired: 2 in, 2 out]
                }
                frame True {
                  n146 = property on="rep time" class="DigNum (strict)"("DisabledEnum"=i8 0) -> ()  [unwired: 2 in, 2 out]
                }
              }
              n147 = property on="exposuretime[ms]" class="DigNum (strict)"("DisabledEnum"=i8 0) -> ()  [unwired: 2 in, 2 out]
            }
            frame Default {
              n148 = global read "Globals.vi" "mshut"() -> (w153:bool)
              n149 = case shown="False" w153 {
                frame False {
                  n150 = property on="exposuretime[ms]" class="DigNum (strict)"("DisabledEnum"=i8 2) -> ()  [unwired: 2 in, 2 out]
                }
                frame True {
                  n151 = property on="exposuretime[ms]" class="DigNum (strict)"("DisabledEnum"=i8 0) -> ()  [unwired: 2 in, 2 out]
                }
              }
              n152 = property on="rep time" class="DigNum (strict)"("DisabledEnum"=i8 2) -> ()  [unwired: 2 in, 2 out]
            }
          }
          n153 = property on="ext. trig. slope" class="RadioBtnsControl (strict)"("DisabledEnum"=w136) -> ()  [unwired: 2 in, 2 out]
          n154 = property on="Scan Trig Input Sel" class="CmbBox"("DisabledEnum"=w136) -> ()  [unwired: 2 in, 2 out]
          n155 = property on="cool" class="DigNum (strict)"("DisabledEnum"=w136) -> ()  [unwired: 2 in, 2 out]
          n156 = property on="BlockSyncStart" class="CmbBox"("DisabledEnum"=w136) -> ()  [unwired: 2 in, 2 out]
          n157 = property on="Board select" class="CmbBox"("DisabledEnum"=w136) -> ()  [unwired: 2 in, 2 out]
          n158 = property on="is FFT" class="Bool (strict)"("DisabledEnum"=w136) -> ()  [unwired: 2 in, 2 out]
          n159 = property on="FFT mode" class="CmbBox"("DisabledEnum"=w136) -> ()  [unwired: 2 in, 2 out]
          n160 = property on="Initialize" class="Bool (strict)"("DisabledEnum"=w136) -> ()  [unwired: 2 in, 2 out]
          n161 = property on="Gain" class="Bool (strict)"("DisabledEnum"=w136) -> ()  [unwired: 2 in, 2 out]
          n162 = property on="fast test\ncontinuous" class="Bool (strict)"("Value"=FALSE) -> ()  [unwired: 2 in, 2 out]
        }
        frame #5 {
          # "xckdelay"
          # "init Board/s"
          # "A/D: 2=8bit, 1=12/16bit"
          n163 = global read "Globals.vi" "CAMCNT"() -> (w169:u32)
          n164 = global read "Globals.vi" "PIXEL"() -> (w171:u32)
          n165 = global read "Globals.vi" "board_sel"() -> (w168:u32)
          n166 = call "InitBrd_multicam.vi"("xckdly"=u32 0, "camcnt"=w169, "pixel"=w171, "board_sel"=w168) -> ()  [unwired: 2 in]
        }
        frame #6 {
          # "select trigger slope"
          n167 = case shown="\"3\"" "ext. trig. slope" {
            frame "1" {
              # "pos. slope"
              n168 = global read "Globals.vi" "board_sel"() -> (w173:u32)
              n169 = call "HiSlope_thread.vi"("board_sel"=w173) -> ()  [unwired: 1 in]
            }
            frame "2" {
              # "neg. slope"
              n170 = global read "Globals.vi" "board_sel"() -> (w174:u32)
              n171 = call "LowSlope_thread.vi"("board_sel"=w174) -> ()  [unwired: 1 in]
            }
            frame "3" {
              # "both slope"
              n172 = global read "Globals.vi" "board_sel"() -> (w175:u32)
              n173 = call "BothSlopes_thread.vi"("board_sel"=w175) -> ()  [unwired: 1 in]
            }
          }
        }
        frame #7 {
          # "if (fkt==0)set to XCK -> XCK\nif (fkt==1)set to REG -> OutTrig\nif (fkt==2)set to CNT_O\nif (fkt==3)set to XCKDLY\nif (fkt==4)set to FFREAD\nif (fkt==5)set to INTTRIG\nif (fkt==6)set to DAT\nif (fkt==7)set to BlockTrig\nif (fkt==8)set to INTRSR\nif (fkt==9)set to S1\nif (fkt==10)set to S2\nif (fkt==11)set to BlockOn\nif (fkt==12)set to MeasureOn\nif (fkt==13)set to XCKDLYON \nif (fkt==14)set to VON         \nif (fkt==15)set to MSHUT"
          # "set TrigOut plug to show:"
          n174 = global read "Globals.vi" "board_sel"() -> (w176:u32)
          n175 = call "SetTOREG_thread.vi"("board_sel"=w176, "fkt"=u8 3) -> ()  [unwired: 1 in]
        }
        frame #8 {
          # "For PDAs S390x"
          # "For IRs G11608"
          # "For PDAs S390x"
          # "For IRs G11608"
          # "register address SEN_GAIN"
          # "implementing FFTs VCLKs"
          n176 = Not(x="is FFT") -> (.not. x?=w183:bool)
          n177 = Boolean To (0,1)(Boolean=w183) -> (0, 1=w184:i16)
          n178 = Boolean To (0,1)(Boolean="Gain") -> (0, 1=w180:i16)
          n179 = To Unsigned Byte Integer(number=w184) -> (unsigned 8bit integer=w181:u8)
          n180 = global read "Globals.vi" "maddr of CAM"() -> (w187:u8)
          n181 = To Unsigned Word Integer(number=w180) -> (unsigned 16bit integer=w178:u16)
          n182 = global read "Globals.vi" "board_sel"() -> (w186:u32)
          n183 = global read "Globals.vi" "board_sel"() -> (w182:u32)
          n184 = call "SendFLCam.vi"("adadr"=u8 0, "data"=w178, "madr"=w187, "board_sel"=w186) -> ()
          n185 = call "SetPDAnotFFT.vi"("set"=w181, "board_sel"=w182) -> ()  [unwired: 1 in]
        }
        frame #9 {
          # "set cooling level"
          n186 = global read "Globals.vi" "CoolCam"() -> (w189:bool)
          n187 = case shown="True" w189 {
            frame False {
            }
            frame True {
              n188 = call "SetTemp.vi"("level 0..7"="cool") -> ()  [unwired: 1 in]
            }
          }
        }
        frame #10 {
          n189 = call "InitProDLL.vi"() -> ()  [unwired: 5 in]
        }
        frame #11 {
          # "for FFT"
          # "register address LED OFF"
          # "select LED OFF\nTrue for LED on\nFalse for LED off"
          n190 = global read "Globals.vi" "LED off"() -> (w191:bool)
          n191 = property on="is FFT" class="Bool (strict)"() -> ("Value"=w194:bool)  [unwired: 2 in, 2 out]
          n192 = global read "Globals.vi" "maddr of CAM"() -> (w197:u8)
          n193 = case shown="True" w194 {
            frame False {
              w219 = u8 44 items=["S0Addr_CtrlA"=4, "S0Addr_CtrlB"=5, "S0Addr_CtrlC"=6, "S0Addr_XCKLL"=8, "S0Addr_XCKLH"=9, "S0Addr_XCKHL"=10, "S0Addr_XCKMSB"=11, "S0Addr_XCKCNTLL"=12, "S0Addr_XCKCNTLH"=13, "S0Addr_XCKCNTHL"=14, "S0Addr_XCKCNTMSB"=15, "S0Addr_PIXREGlow"=16, "S0Addr_PIXREGhigh"=17, "S0Addr_FREQREG"=18, "S0Addr_FF_FLAGS"=19, "S0Addr_FIFOCNT"=20, "S0Addr_VCLKCTRL"=24, "S0Addr_EBST"=28, "S0Addr_DAT"=32, "S0Addr_EC"=36, "S0Addr_TOR"=40, "S0Addr_ARREG"=44, "S0Addr_GIOREG"=48, "S0Addr_DELAYEC"=52, "S0Addr_IRQREG"=56, "S0Addr_PCI"=60]
              # "turn partial binning off"
              n194 = call "WriteL.vi"("val"=u32 0, "offset"=w219) -> ()
            }
            frame True {
              n195 = case shown="\"Full Binning\", Default" "FFT mode" {
                frame "Full Binning", Default {
                  # "only needed for FFTs"
                  # "lines = vclks"
                  n196 = global read "Globals.vi" "board_sel"() -> (w224:u32)
                  n197 = global read "Globals.vi" "vfreq"() -> (w222:u8)
                  n198 = global read "Globals.vi" "lines"() -> (w223:u32)
                  n199 = call "SetupFullBinning.vi"("vfreq"=w222, "lines"=w223, "drvno"=w224) -> ()
                }
                frame "Area" {
                  # "only needed for FFTs"
                  # "lines = vclks"
                  n200 = global read "Globals.vi" "area_lines_binning"() -> (w227:u32)
                  n201 = global read "Globals.vi" "vfreq"() -> (w225:u8)
                  n202 = global read "Globals.vi" "board_sel"() -> (w226:u32)
                  n203 = global read "Globals.vi" "area_lines_binning"() -> (w230:u32)
                  n204 = global read "Globals.vi" "lines"() -> (w231:u32)
                  n205 = call "SetupArea.vi"("vfreq"=w225, "lines_binning"=w227, "drvno"=w226) -> ()
                  n206 = Divide(x=w231, y=w230) -> (x/y=w228:dbl)
                  n207 = To Unsigned Long Integer(number=w228) -> (unsigned 32bit integer=w229:u32)
                  n208 = property on="no.of samples (nos)" class="DigNum (strict)"("Value"=w229) -> ()  [unwired: 2 in, 2 out]
                }
                frame "Region of Interest" {
                  n209 = global read "Globals.vi" "board_sel"() -> (w239:u32)
                  n210 = global read "Globals.vi" "region_size"() -> (w234:u8[])
                  n211 = global read "Globals.vi" "nor"() -> (w236:u32)
                  n212 = global read "Globals.vi" "lines"() -> (w238:u32)
                  n213 = To Unsigned Word Integer(number=w236) -> (unsigned 16bit integer=w237:u16)
                  n214 = call "SetupROI.vi"("keep_first"=u8 0, "vfreq"=u8 7, "region_size"=w234, "lines"=w238, "number_of_regions"=w237, "drv"=w239) -> ()
                  n215 = global read "Globals.vi" "nor"() -> (w232:u32)
                  n216 = property on="no.of samples (nos)" class="DigNum (strict)"("Value"=w232) -> ()  [unwired: 2 in, 2 out]
                }
              }
            }
          }
          n217 = case shown="\"I\", Default" "Scan Trig Input Sel" {
            frame "S1" {
              w206 = u8 5 items=["S0Addr_CtrlA"=4, "S0Addr_CtrlB"=5, "S0Addr_CtrlC"=6, "S0Addr_XCKLL"=8, "S0Addr_XCKLH"=9, "S0Addr_XCKHL"=10, "S0Addr_XCKMSB"=11, "S0Addr_XCKCNTLL"=12, "S0Addr_XCKCNTLH"=13, "S0Addr_XCKCNTHL"=14, "S0Addr_XCKCNTMSB"=15, "S0Addr_PIXREGlow"=16, "S0Addr_PIXREGhigh"=17, "S0Addr_FREQREG"=18, "S0Addr_FF_FLAGS"=19, "S0Addr_FIFOCNT"=20, "S0Addr_VCLKCTRL"=24, "S0Addr_EBST"=28, "S0Addr_DAT"=32, "S0Addr_EC"=36, "S0Addr_TOR"=40, "S0Addr_ARREG"=44, "S0Addr_GIOREG"=48, "S0Addr_DELAYEC"=52, "S0Addr_IRQREG"=56, "S0Addr_PCI"=60]
              w201 = u8 5 items=["S0Addr_CtrlA"=4, "S0Addr_CtrlB"=5, "S0Addr_CtrlC"=6, "S0Addr_XCKLL"=8, "S0Addr_XCKLH"=9, "S0Addr_XCKHL"=10, "S0Addr_XCKMSB"=11, "S0Addr_XCKCNTLL"=12, "S0Addr_XCKCNTLH"=13, "S0Addr_XCKCNTHL"=14, "S0Addr_XCKCNTMSB"=15, "S0Addr_PIXREGlow"=16, "S0Addr_PIXREGhigh"=17, "S0Addr_FREQREG"=18, "S0Addr_FF_FLAGS"=19, "S0Addr_FIFOCNT"=20, "S0Addr_VCLKCTRL"=24, "S0Addr_EBST"=28, "S0Addr_DAT"=32, "S0Addr_EC"=36, "S0Addr_TOR"=40, "S0Addr_ARREG"=44, "S0Addr_GIOREG"=48, "S0Addr_DELAYEC"=52, "S0Addr_IRQREG"=56, "S0Addr_PCI"=60]
              # "Trig in: S1"
              n218 = global read "Globals.vi" "board_sel"() -> (w202:u32)
              n219 = call "ResetS0Bit.vi"("drv"=w202, "Address"=w201, "bitnumber"=u32 5) -> ()
              n220 = global read "Globals.vi" "board_sel"() -> (w205:u32)
              n221 = call "SetS0Bit.vi"("board_sel"=w205, "Address"=w206, "bitnumber"=u32 4) -> ()
            }
            frame "S2" {
              w207 = u8 5 items=["S0Addr_CtrlA"=4, "S0Addr_CtrlB"=5, "S0Addr_CtrlC"=6, "S0Addr_XCKLL"=8, "S0Addr_XCKLH"=9, "S0Addr_XCKHL"=10, "S0Addr_XCKMSB"=11, "S0Addr_XCKCNTLL"=12, "S0Addr_XCKCNTLH"=13, "S0Addr_XCKCNTHL"=14, "S0Addr_XCKCNTMSB"=15, "S0Addr_PIXREGlow"=16, "S0Addr_PIXREGhigh"=17, "S0Addr_FREQREG"=18, "S0Addr_FF_FLAGS"=19, "S0Addr_FIFOCNT"=20, "S0Addr_VCLKCTRL"=24, "S0Addr_EBST"=28, "S0Addr_DAT"=32, "S0Addr_EC"=36, "S0Addr_TOR"=40, "S0Addr_ARREG"=44, "S0Addr_GIOREG"=48, "S0Addr_DELAYEC"=52, "S0Addr_IRQREG"=56, "S0Addr_PCI"=60]
              w210 = u8 5 items=["S0Addr_CtrlA"=4, "S0Addr_CtrlB"=5, "S0Addr_CtrlC"=6, "S0Addr_XCKLL"=8, "S0Addr_XCKLH"=9, "S0Addr_XCKHL"=10, "S0Addr_XCKMSB"=11, "S0Addr_XCKCNTLL"=12, "S0Addr_XCKCNTLH"=13, "S0Addr_XCKCNTHL"=14, "S0Addr_XCKCNTMSB"=15, "S0Addr_PIXREGlow"=16, "S0Addr_PIXREGhigh"=17, "S0Addr_FREQREG"=18, "S0Addr_FF_FLAGS"=19, "S0Addr_FIFOCNT"=20, "S0Addr_VCLKCTRL"=24, "S0Addr_EBST"=28, "S0Addr_DAT"=32, "S0Addr_EC"=36, "S0Addr_TOR"=40, "S0Addr_ARREG"=44, "S0Addr_GIOREG"=48, "S0Addr_DELAYEC"=52, "S0Addr_IRQREG"=56, "S0Addr_PCI"=60]
              # "Trig in: S2"
              n222 = global read "Globals.vi" "board_sel"() -> (w211:u32)
              n223 = call "SetS0Bit.vi"("board_sel"=w211, "Address"=w210, "bitnumber"=u32 5) -> ()
              n224 = global read "Globals.vi" "board_sel"() -> (w208:u32)
              n225 = call "ResetS0Bit.vi"("drv"=w208, "Address"=w207, "bitnumber"=u32 4) -> ()
            }
            frame "I", Default {
              w218 = u8 5 items=["S0Addr_CtrlA"=4, "S0Addr_CtrlB"=5, "S0Addr_CtrlC"=6, "S0Addr_XCKLL"=8, "S0Addr_XCKLH"=9, "S0Addr_XCKHL"=10, "S0Addr_XCKMSB"=11, "S0Addr_XCKCNTLL"=12, "S0Addr_XCKCNTLH"=13, "S0Addr_XCKCNTHL"=14, "S0Addr_XCKCNTMSB"=15, "S0Addr_PIXREGlow"=16, "S0Addr_PIXREGhigh"=17, "S0Addr_BTRIGREG"=18, "S0Addr_FF_FLAGS"=19, "S0Addr_FIFOCNT"=20, "S0Addr_VCLKCTRL"=24, "S0Addr_EBST"=28, "S0Addr_DAT"=32, "S0Addr_EC"=36, "S0Addr_TOR"=40, "S0Addr_ARREG"=44, "S0Addr_GIOREG"=48, "S0Addr_DELAYEC"=52, "S0Addr_IRQREG"=56, "S0Addr_PCI"=60]
              w213 = u8 5 items=["S0Addr_CtrlA"=4, "S0Addr_CtrlB"=5, "S0Addr_CtrlC"=6, "S0Addr_XCKLL"=8, "S0Addr_XCKLH"=9, "S0Addr_XCKHL"=10, "S0Addr_XCKMSB"=11, "S0Addr_XCKCNTLL"=12, "S0Addr_XCKCNTLH"=13, "S0Addr_XCKCNTHL"=14, "S0Addr_XCKCNTMSB"=15, "S0Addr_PIXREGlow"=16, "S0Addr_PIXREGhigh"=17, "S0Addr_BTRIGREG"=18, "S0Addr_FF_FLAGS"=19, "S0Addr_FIFOCNT"=20, "S0Addr_VCLKCTRL"=24, "S0Addr_EBST"=28, "S0Addr_DAT"=32, "S0Addr_EC"=36, "S0Addr_TOR"=40, "S0Addr_ARREG"=44, "S0Addr_GIOREG"=48, "S0Addr_DELAYEC"=52, "S0Addr_IRQREG"=56, "S0Addr_PCI"=60]
              # "Trig in: I"
              n226 = global read "Globals.vi" "board_sel"() -> (w217:u32)
              n227 = call "ResetS0Bit.vi"("drv"=w217, "Address"=w218, "bitnumber"=u32 5) -> ()
              n228 = global read "Globals.vi" "board_sel"() -> (w214:u32)
              n229 = call "ResetS0Bit.vi"("drv"=w214, "Address"=w213, "bitnumber"=u32 4) -> ()
            }
          }
          n230 = global read "Globals.vi" "board_sel"() -> (w195:u32)
          n231 = case shown="False" w191 {
            tunnel: [u16 0 u16 1] -> w196
            frame False {
              # "send 1 for LED off"
            }
            frame True {
              # "send 0 for LED on"
            }
          }
          n232 = call "SendFLCam.vi"("adadr"=u8 5, "data"=w196, "madr"=w197, "board_sel"=w195) -> ()
          n233 = global read "Globals.vi" "mshut"() -> (w192:bool)
          n234 = case shown="True" w192 {
            frame False {
            }
            frame True {
              # "Close Shutter"
              n235 = global read "Globals.vi" "board_sel"() -> (w200:u32)
              n236 = property on="shutter open" class="Bool (strict)"("Value"=FALSE) -> ()  [unwired: 2 in, 2 out]
              n237 = call "closeshutter.vi"("board_sel"=w200) -> ()  [unwired: 1 in]
            }
          }
        }
        frame #12 {
          # "set gamma settings for bitmap viewer"
          n238 = global read "Globals.vi" "camera system select"() -> (w242:u8)
          n239 = case shown="1, Default" w242 {
            frame 1, Default {
              n240 = property on="value white" class="DigNum (strict)"("Value"=u32 65535) -> ()  [unwired: 2 in, 2 out]
              n241 = property on="value black" class="DigNum (strict)"("Value"=u32 0) -> ()  [unwired: 2 in, 2 out]
            }
            frame 2 {
              n242 = property on="value black" class="DigNum (strict)"("Value"=u32 0) -> ()  [unwired: 2 in, 2 out]
              n243 = property on="value white" class="DigNum (strict)"("Value"=u32 65535) -> ()  [unwired: 2 in, 2 out]
            }
            frame 3 {
              n244 = property on="value black" class="DigNum (strict)"("Value"=u32 0) -> ()  [unwired: 2 in, 2 out]
              n245 = property on="value white" class="DigNum (strict)"("Value"=u32 16383) -> ()  [unwired: 2 in, 2 out]
            }
          }
        }
        frame #13 {
          n246 = global read "Globals.vi" "use GPX"() -> (w249:bool)
          n247 = case shown="True" w249 {
            frame False {
            }
            frame True {
              n248 = global read "Globals.vi" "GPX Offset"() -> (w250:u32)
              n249 = call "InitGPX.vi"("delay"=w250) -> ()  [unwired: 1 in]
            }
          }
        }
        frame #14 {
          # "BlockSync Start\nthe Input (S1, S2 or S1&S2) for special shutter is only working for full binning"
          n250 = case shown="\"Intern\", Default" "BlockSyncStart" {
            tunnel: [u8 3 u8 4 u8 2 u8 0] -> w251
            frame "S2" {
            }
            frame "S1&S2" {
            }
            frame "S1" {
            }
            frame "Intern", Default {
            }
          }
          n251 = global write "Globals.vi" "block_ch"(w251) -> ()
        }
      }
    }
    frame #2 {
      # "init routines for different camera systems"
      n252 = global read "Globals.vi" "camera system select"() -> (w257:u8)
      n253 = case shown="1" w257 {
        frame 1 {
          w264 = u16 0  # trigger
          # "select VCLK ON\n0 for VCLK off\n1 for VCLK on"
          # "set trigger input\ntrigger = x0 XCK\ntrigger = x1 EXTTRIG\ntrigger = x2 DAT"
          # "init routine for 3001"
          n254 = property on="FFT mode" class="CmbBox"() -> ("Value"=w262:string)  [unwired: 2 in, 2 out]
          n255 = property on="is FFT" class="Bool (strict)"() -> ("Value"=w260:bool)  [unwired: 2 in, 2 out]
          n256 = case shown="\"Area\"" w262 {
            tunnel: [u16 0 w268] -> w261
            frame Default {
            }
            frame "Area" {
              n257 = global read "Globals.vi" "area_lines_binning"() -> (w269:u32)
              n258 = case shown="1" w269 {
                tunnel: [u16 0 u16 1] -> w268
                frame Default {
                }
                frame 1 {
                }
              }
            }
          }
          n259 = global read "Globals.vi" "PIXEL"() -> (w266:u32)
          n260 = global read "Globals.vi" "board_sel"() -> (w265:u32)
          n261 = Boolean To (0,1)(Boolean=w260) -> (0, 1=w259:i16)
          n262 = To Unsigned Word Integer(number=w259) -> (unsigned 16bit integer=w258:u16)
          n263 = To Unsigned Word Integer(number=w266) -> (unsigned 16bit integer=w263:u16)
          n264 = call "InitCam3001.vi"("IS_AREA"=w261, "pixel"=w263, "IS_FFT"=w258, "trigger_input"=w264, "drvno"=w265) -> ()  [unwired: 1 in]
        }
        frame 2 {
          w277 = u8 0  # adc mode
          w278 = u16 0  # trigger input
          w276 = u16 170  # custom pattern
          w275 = u16 0  # led
          # "init routine for 3010"
          # "adc mode = x0 normal\nadc mode = x2 custom pattern"
          # "set trigger input\ntrigger input = x0 XCK\ntrigger input  = x1 EXTTRIG\ntrigger input  = x2 DAT"
          n265 = global read "Globals.vi" "board_sel"() -> (w280:u32)
          n266 = global read "Globals.vi" "PIXEL"() -> (w281:u32)
          n267 = To Unsigned Word Integer(number=w281) -> (unsigned 16bit integer=w279:u16)
          n268 = Boolean To (0,1)(Boolean="camera gain") -> (0, 1=w274:i16)
          n269 = To Unsigned Word Integer(number=w274) -> (unsigned 16bit integer=w272:u16)
          n270 = call "InitCam3010.vi"("gain_high"=w272, "led_on"=w275, "custom_pattern"=w276, "adc_mode"=w277, "trigger_input"=w278, "pixel"=w279, "drvno"=w280) -> ()
        }
        frame 3, Default {
          # "init routine for 3030"
          n271 = flat-sequence {
            frame #0 {
              n272 = case shown="\"1\"" "ADC mode 2" {
                tunnel: [w288 w289 w290] -> w284
                frame "1" {
                  w288 = u8 2  # adc mode
                  # "Custom Pattern"
                }
                frame "2" {
                  w289 = u8 1  # adc mode
                  # "Ramp"
                }
                frame "3" {
                  w290 = u8 0  # adc mode
                  # "Normal Mode"
                }
              }
              n273 = global read "Globals.vi" "cam gain"() -> (w286:u32)
              n274 = global read "Globals.vi" "board_sel"() -> (w285:u32)
              n275 = To Unsigned Byte Integer(number=w286) -> (unsigned 8bit integer=w282:u8)
              n276 = call "InitCam3030.vi"("gain_high"=w282, "custom_pattern"="pattern hex (2)", "adc_mode"=w284, "drvno"=w285) -> ()  [unwired: 1 in]
              "pattern dec 2" <- "pattern hex (2)"
            }
            frame #1 {
              # "EN DAC internal ref.\nPCB 2189-7 only"
              n277 = global read "Globals.vi" "use DAC"() -> (w291:bool)
              n278 = case shown="True" w291 {
                frame False {
                }
                frame True {
                  w292 = u16 0  # data (hex)
                  w297 = u8 1  # feature (hex)
                  w296 = u8 0  # addr (hex)
                  w295 = u8 8  # ctrl (hex)
                  n279 = global read "Globals.vi" "board_sel"() -> (w294:u32)
                  n280 = To Unsigned Byte Integer(number=w297) -> (unsigned 8bit integer=w298:u8)
                  n281 = To Unsigned Byte Integer(number=w296) -> (unsigned 8bit integer=w299:u8)
                  n282 = To Unsigned Byte Integer(number=w295) -> (unsigned 8bit integer=w293:u8)
                  n283 = call "SendFLCam_DAC.vi"("board_sel"=w294, "ctrl"=w293, "feature"=w298, "data"=w292, "addr"=w299) -> ()
                }
              }
            }
          }
        }
      }
    }
    frame #3 {
      w302 = FALSE
      w304 = 2
      # "cosmetics of the graphs for more cams"
      n284 = property on="framewise\ncontinuous" class="Bool (strict)"("DisabledEnum"=w304) -> ()  [unwired: 2 in, 2 out]
      n285 = property on="block" class="Slide (strict)"("DisabledEnum"=w304) -> ()  [unwired: 2 in, 2 out]
      n286 = property on="fast test\ncontinuous" class="Bool (strict)"("DisabledEnum"=w304) -> ()  [unwired: 2 in, 2 out]
      n287 = property on="start" class="Bool (strict)"("DisabledEnum"=w304) -> ()  [unwired: 2 in, 2 out]
      n288 = property on="sample" class="Slide (strict)"("DisabledEnum"=w304) -> ()  [unwired: 2 in, 2 out]
      n289 = property on="stop all" class="Bool (strict)"("DisabledEnum"=0) -> ()  [unwired: 2 in, 2 out]
      n290 = Boolean To (0,1)(Boolean=w302) -> (0, 1=w301:i16)
      n291 = property on="Measure ON" class="Bool (strict)"("Value"=w302) -> ()  [unwired: 2 in, 2 out]
      n292 = To Unsigned Byte Integer(number=w301) -> (unsigned 8bit integer=w300:u8)
      n293 = property on="framewise\ncontinuous" class="Bool (strict)"("Value"=w302) -> ()  [unwired: 2 in, 2 out]
      n294 = call "contFFLoop.vi"("Numeric"=w300) -> ()  [unwired: 1 in]
      n295 = global read "Globals.vi" "boards"() -> (w303:u32)
      n296 = case shown="2" w303 {
        frame 2 {
          n297 = global read "Globals.vi" "CAMCNT"() -> (w310:u32)
          n298 = case shown="1, Default" w310 {
            tunnel: [TRUE w317 w318 w320] -> w309
            tunnel: [w314 w317 w318 w320] -> w308
            tunnel: [w314 FALSE w318 w320] -> w307
            frame 2 {
              w314 = FALSE
              n299 = property on="Signal Board 1 / Cam 1" class="WFGraph (strict)"("Height"=u32 170) -> ()  [unwired: 2 in, 2 out]
            }
            frame 3 {
              w317 = TRUE
            }
            frame 4 {
              w318 = TRUE
            }
            frame 1, Default {
              w320 = FALSE
              n300 = property on="Signal Board 1 / Cam 1" class="WFGraph (strict)"("Height"=u32 170) -> ()  [unwired: 2 in, 2 out]
              n301 = property on="Signal Board 1 / Cam1" class="WFGraph (strict)"("Top"=0) -> ()  [unwired: 2 in, 2 out]
            }
          }
          n302 = property on="Signal Board 1 / Cam1" class="WFGraph (strict)"("Height"=u32 170) -> ()  [unwired: 2 in, 2 out]
          n303 = property on="Signal Board 2 / Cam1" class="WFGraph (strict)"("Visible"=TRUE) -> ()  [unwired: 2 in, 2 out]
          n304 = property on="Signal Board 1 / Cam 3" class="WFGraph (strict)"("Visible"=w308) -> ()  [unwired: 2 in, 2 out]
          n305 = property on="Signal Board 1 / Cam 4" class="WFGraph (strict)"("Visible"=w307) -> ()  [unwired: 2 in, 2 out]
          n306 = property on="Signal Board 1 / Cam 2" class="WFGraph (strict)"("Visible"=w309) -> ()  [unwired: 2 in, 2 out]
        }
        frame 1, Default {
          n307 = global read "Globals.vi" "CAMCNT"() -> (w325:u32)
          n308 = case shown="2" w325 {
            tunnel: [TRUE w335 w340 w341] -> w324
            tunnel: [w329 w335 w340 w341] -> w323
            tunnel: [w329 FALSE w340 w341] -> w322
            frame 2 {
              w329 = FALSE
              n309 = property on="Signal Board 1 / Cam1" class="WFGraph (strict)"("Height"=u32 170) -> ()  [unwired: 2 in, 2 out]
              n310 = property on="Signal Cam 2" class="WFGraph (strict)"("Top"=250) -> ()  [unwired: 2 in, 2 out]
            }
            frame 3 {
              w335 = TRUE
              n311 = property on="Signal Board 1 / Cam1" class="WFGraph (strict)"("Height"=u32 170) -> ()  [unwired: 2 in, 2 out]
              n312 = property on="Signal Cam 2" class="WFGraph (strict)"("Top"=250) -> ()  [unwired: 2 in, 2 out]
              n313 = property on="Signal Cam 3" class="WFGraph (strict)"("Top"=-250) -> ()  [unwired: 2 in, 2 out]
            }
            frame 4 {
              w340 = TRUE
              n314 = property on="Signal Board 1 / Cam1" class="WFGraph (strict)"("Height"=u32 170) -> ()  [unwired: 2 in, 2 out]
              n315 = property on="Signal Cam 3" class="WFGraph (strict)"("Top"=-250) -> ()  [unwired: 2 in, 2 out]
              n316 = property on="Signal Cam 2" class="WFGraph (strict)"("Top"=250) -> ()  [unwired: 2 in, 2 out]
              n317 = property on="Signal Cam 4" class="WFGraph (strict)"("Top"=-500) -> ()  [unwired: 2 in, 2 out]
            }
            frame 1, Default {
              w341 = FALSE
              n318 = property on="Signal Board 1 / Cam1" class="WFGraph (strict)"("Height"=u32 400) -> ()  [unwired: 2 in, 2 out]
            }
          }
          n319 = property on="Signal Board 2 / Cam1" class="WFGraph (strict)"("Visible"=FALSE) -> ()  [unwired: 2 in, 2 out]
          n320 = property on="Signal Cam 3" class="WFGraph (strict)"("Visible"=w323) -> ()  [unwired: 2 in, 2 out]
          n321 = property on="Signal Cam 4" class="WFGraph (strict)"("Visible"=w322) -> ()  [unwired: 2 in, 2 out]
          n322 = property on="Signal Cam 2" class="WFGraph (strict)"("Visible"=w324) -> ()  [unwired: 2 in, 2 out]
        }
      }
      n323 = property on="# boards \ndetected" class="DigNum (strict)"("Visible"=TRUE) -> ()  [unwired: 2 in, 2 out]
    }
    frame #4 {
      # "display / hide chosen labview elements"
      n324 = global read "Globals.vi" "debug_mode"() -> (w350:bool)
      n325 = global read "Globals.vi" "camera system select"() -> (w346:u8)
      n326 = case shown="3" w346 {
        tunnel: [FALSE FALSE TRUE] -> w347
        frame 1, Default {
        }
        frame 2 {
        }
        frame 3 {
        }
      }
      n327 = And(x=w347, y=w350) -> (x .and. y?=w344:bool)
      n328 = property on="custom patt: 14bits pattern hex (14bit)" class="DigNum (strict)"("Visible"=w344) -> ()  [unwired: 2 in, 2 out]
      n329 = property on="ADC mode" class="RadioBtnsControl (strict)"("Visible"=w344) -> ()  [unwired: 2 in, 2 out]
      n330 = property on="pattern dec" class="DigNum (strict)"("Visible"=w344) -> ()  [unwired: 2 in, 2 out]
      n331 = case shown="2" w346 {
        tunnel: [FALSE TRUE FALSE] -> w348
        frame 1, Default {
        }
        frame 2 {
        }
        frame 3 {
        }
      }
      n332 = property on="camera gain" class="Bool (strict)"("Visible"=w348) -> ()  [unwired: 2 in, 2 out]
      n333 = global read "Globals.vi" "use DAC"() -> (w349:bool)
      n334 = And(x=w347, y=w349) -> (x .and. y?=w343:bool)
      n335 = property on="DAC 3/ 1" class="DigNum (strict)"("Visible"=w343) -> ()  [unwired: 2 in, 2 out]
      n336 = property on="DAC 5/ 1" class="DigNum (strict)"("Visible"=w343) -> ()  [unwired: 2 in, 2 out]
      n337 = property on="DAC 4/ 1" class="DigNum (strict)"("Visible"=w343) -> ()  [unwired: 2 in, 2 out]
      n338 = property on="DAC 6/ 1" class="DigNum (strict)"("Visible"=w343) -> ()  [unwired: 2 in, 2 out]
      n339 = property on="DAC 7/ 1" class="DigNum (strict)"("Visible"=w343) -> ()  [unwired: 2 in, 2 out]
      n340 = property on="DAC 8/ 1" class="DigNum (strict)"("Visible"=w343) -> ()  [unwired: 2 in, 2 out]
      n341 = property on="DAC 1/ 1" class="DigNum (strict)"("Visible"=w343) -> ()  [unwired: 2 in, 2 out]
      n342 = property on="Offset" class="Bool (strict)"("Visible"=w343) -> ()  [unwired: 2 in, 2 out]
      n343 = property on="DAC 2/ 1" class="DigNum (strict)"("Visible"=w343) -> ()  [unwired: 2 in, 2 out]
      n344 = property on="Offset" class="Bool (strict)"() -> ("Value"=w345:bool)  [unwired: 2 in, 2 out]
      n345 = property on="Offset" class="Bool (strict)"("Val(Sgnl)"=w345) -> ()  [unwired: 2 in, 2 out]
    }
    frame #5 {
      # "event structure while running"
      n346 = while {
        stop <- w358 stop-if-true
        n347 = event shown="[7] \"startevent\": Value Change" {
          selector: _ -> [_ _ _ _ _ _ _ _ _ _ _ _ _ _ _ _ _ _ _ _ _ _ _]
          dyn-events: _ -> [_ _ _ _ _ _ _ _ _ _ _ _ _ _ _ _ _ _ _ _ _ _ _]
          timeout: 100 -> [_ _ _ _ _ _ _ _ _ _ _ _ _ _ _ _ _ _ _ _ _ _ _]
          tunnel: [_ _ _ _ _ _ _ _ _ _ _ _ _ _ w715 _ _ _ _ _ _ _ _] -> w358
          event Timeout; "refresh": Value Change {
            w364 = u32 0
            w387 = u32 1
            # "only refresh the frames if measure on"
            # "compares measure on signal from hardware with measure on lamp\nwhen diffrent than write new measure on value to lamp"
            # "timout excecutes every 100ms"
            # "userinfo of RAM, MeasureOB, Curr.Block and setting display event in cont mode"
            n348 = event-data() -> ()  [unwired: 1 in, 3 out]
            n349 = call "FreeMemInfo.vi"() -> ("PhysicalSpace"=→"BUILT-IN\nRAM MB":dbl, "PhysicalFreeSpace"=→"FREE \nRAM MB":dbl)  [unwired: 1 in]
            n350 = property on="framewise\ncontinuous" class="Bool (strict)"() -> ("DisabledEnum"=w397:T1)  [unwired: 2 in, 2 out]
            n351 = global read "Globals.vi" "board_sel"() -> (w360:u32)
            n352 = global read "Globals.vi" "nos"() -> (w388:u32)
            n353 = global read "Globals.vi" "nob"() -> (w389:u32)
            n354 = property on="Measure ON" class="Bool (strict)"() -> ("Value"=w401:bool)  [unwired: 2 in, 2 out]
            n355 = property on="framewise\ncontinuous" class="Bool (strict)"() -> ("Value"=w363:bool)  [unwired: 2 in, 2 out]
            n356 = call "isMeasureOn.vi"("drv"=w360) -> ("Measure On"=w359:bool)
            n357 = Not Equal?(x=w401, y=w359) -> (x != y?=w400:bool)
            n358 = Equal?(x=w389, y=w387) -> (x = y?=w385:bool)
            n359 = Equal?(x=w387, y=w388) -> (x = y?=w386:bool)
            n360 = To Unsigned Byte Integer(number=w397) -> (unsigned 8bit integer=w398:u8)
            n361 = And(x=w385, y=w386) -> (x .and. y?=w384:bool)
            n362 = Equal?(x=w398, y=u8 0) -> (x = y?=w362:bool)
            n363 = global read "Globals.vi" "board_sel"() -> (w365:u32)
            n364 = case shown="True" w400 {
              tunnel: w359 -> [_ w408]
              frame False {
              }
              frame True {
                n365 = property on="Measure ON" class="Bool (strict)"("Val(Sgnl)"=w408) -> ()  [unwired: 2 in, 2 out]
              }
            }
            n366 = call "BitTest.vi"("BitAddr"=u32 8, "Offset"=w364, "board_sel"=w365) -> ("Bool Board 1"=→"(LastCAM) \n        C1":bool)  [unwired: 1 out]
            n367 = call "BitTest.vi"("BitAddr"=u32 9, "Offset"=w364, "board_sel"=w365) -> ("Bool Board 1"=→"C 2":bool)  [unwired: 1 out]
            n368 = call "BitTest.vi"("BitAddr"=u32 10, "Offset"=w364, "board_sel"=w365) -> ("Bool Board 1"=→"C 3":bool)  [unwired: 1 out]
            n369 = call "BitTest.vi"("BitAddr"=u32 11, "Offset"=w364, "board_sel"=w365) -> ("Bool Board 1"=→"C 4":bool)  [unwired: 1 out]
            n370 = global read "Globals.vi" "board_sel"() -> (w383:u32)
            n371 = And(x=w363, y=w362) -> (x .and. y?=w391:bool)
            n372 = Or(x=w384, y=w391) -> (x .or. y?=w390:bool)
            n373 = call "ReadL.vi"("Offset"=w364, "board_sel"=w365) -> ("Data 1"=→"cool_temp Reg":u32)  [unwired: 1 out]
            n374 = And(x=w390, y=w359) -> (x .and. y?=w392:bool)
            n375 = call "ReadB.vi"("Offset"=u32 88, "board_sel"=w383) -> ("Data 2"=w393:u8, "Data 1"=w394:u8)
            n376 = call "BitTest.vi"("BitAddr"=u32 12, "Offset"=w364, "board_sel"=w365) -> ("Bool Board 1"=→"C 5":bool)  [unwired: 1 out]
            n377 = call "BitTest.vi"("BitAddr"=u32 13, "Offset"=w364, "board_sel"=w365) -> ("Bool Board 1"=→"C 6":bool)  [unwired: 1 out]
            n378 = call "BitTest.vi"("BitAddr"=u32 14, "Offset"=w364, "board_sel"=w365) -> ("Bool Board 1"=→"C 7":bool)  [unwired: 1 out]
            n379 = call "BitTest.vi"("BitAddr"=u32 15, "Offset"=w364, "board_sel"=w365) -> ("Bool Board 1"=→"C 8":bool)  [unwired: 1 out]
            n380 = case shown="True" w392 {
              frame False {
              }
              frame True {
                # "trigger the \ndisplay event"
                n381 = property on="sample" class="Slide (strict)"() -> ("Value"=w409:u32)  [unwired: 2 in, 2 out]
                n382 = property on="sample" class="Slide (strict)"("Val(Sgnl)"=w409) -> ()  [unwired: 2 in, 2 out]
              }
            }
            n383 = case shown="True" w359 {
              tunnel: [2 0] -> w361
              frame False {
              }
              frame True {
              }
            }
            n384 = case shown="2" w383 {
              tunnel: [w406 w407] -> w395
              tunnel: w394 -> [_ w407]
              tunnel: w393 -> [w406 _]
              frame 2 {
              }
              frame 1, 3, Default {
              }
            }
            "curr_read_block" <- w395
            n385 = property on="(LastCAM) \n        C1" class="Bool (strict)"("DisabledEnum"=w361) -> ()  [unwired: 2 in, 2 out]
            n386 = property on="C 2" class="Bool (strict)"("DisabledEnum"=w361) -> ()  [unwired: 2 in, 2 out]
            n387 = property on="C 3" class="Bool (strict)"("DisabledEnum"=w361) -> ()  [unwired: 2 in, 2 out]
            n388 = property on="C 4" class="Bool (strict)"("DisabledEnum"=w361) -> ()  [unwired: 2 in, 2 out]
            n389 = property on="C 5" class="Bool (strict)"("DisabledEnum"=w361) -> ()  [unwired: 2 in, 2 out]
            n390 = property on="C 6" class="Bool (strict)"("DisabledEnum"=w361) -> ()  [unwired: 2 in, 2 out]
            n391 = property on="C 7" class="Bool (strict)"("DisabledEnum"=w361) -> ()  [unwired: 2 in, 2 out]
            n392 = property on="C 8" class="Bool (strict)"("DisabledEnum"=w361) -> ()  [unwired: 2 in, 2 out]
          }
          event "Measure ON": Value Change {
            # "triggers on value change of measure on. this happens on start of measurement and after measurement\nwhen continuous: not after finishing all blocks, only when exiting measurement"
            n393 = event-data() -> ("NewVal"=w410:bool)  [unwired: 1 in, 5 out]
            n394 = case shown="True" w410 {
              tunnel: w410 -> [_ w411]
              frame False {
              }
              frame True {
                n395 = flat-sequence {
                  tunnel: w411 -> [w412]
                  frame #0 {
                    n396 = property on="fast test\ncontinuous" class="Bool (strict)"() -> ("Value"=w416:bool)  [unwired: 2 in, 2 out]
                    n397 = property on="framewise\ncontinuous" class="Bool (strict)"() -> ("Value"=w415:bool)  [unwired: 2 in, 2 out]
                    n398 = Or(x=w415, y=w416) -> (x .or. y?=w414:bool)
                    n399 = And(x=w414, y=w412) -> (x .and. y?=w413:bool)
                    n400 = case shown="True" w413 {
                      frame False {
                      }
                      frame True {
                        n401 = property on="stop all" class="Bool (strict)"("DisabledEnum"=2) -> ()  [unwired: 2 in, 2 out]
                      }
                    }
                  }
                  frame #1 {
                    # "wait until end\nof measurement"
                    n402 = global read "Globals.vi" "board_sel"() -> (w418:u32)
                    n403 = call "waitForMeasureReady.vi"("drv"=w418) -> ()
                  }
                  frame #2 {
                    # "end of measuring"
                    n404 = property on="TRMS Pix" class="DigNum (strict)"() -> ("Value"=w420:u32)  [unwired: 2 in, 2 out]
                    n405 = property on="sample" class="Slide (strict)"() -> ("Value"=w421:u32)  [unwired: 2 in, 2 out]
                    n406 = property on="TRMS Pix" class="DigNum (strict)"("Val(Sgnl)"=w420) -> ()  [unwired: 2 in, 2 out]
                    n407 = property on="sample" class="Slide (strict)"("Val(Sgnl)"=w421) -> ()  [unwired: 2 in, 2 out]
                    n408 = property on="stop all" class="Bool (strict)"("DisabledEnum"=0) -> ()  [unwired: 2 in, 2 out]
                  }
                  frame #3 {
                    # "Do math here"
                  }
                }
              }
            }
          }
          event "framewise\ncontinuous": Value Change {
            n409 = event-data() -> ()  [unwired: 1 in, 6 out]
            n410 = property on="is FFT" class="Bool (strict)"() -> ("Value"=w432:bool)  [unwired: 2 in, 2 out]
            n411 = case shown="True" "framewise\ncontinuous" {
              tunnel: [u8 0 u8 1] -> w434
              tunnel: [u8 2 u8 0] -> w433
              tunnel: [FALSE FALSE] -> w430
              tunnel: [u8 0 w448] -> w431
              frame False {
              }
              frame True {
                n412 = property on="sample" class="Slide (strict)"() -> ("DisabledEnum"=w448:T1)  [unwired: 2 in, 2 out]
              }
            }
            n413 = property on="no.of blocks (nob)" class="DigNum (strict)"("DisabledEnum"=w431) -> ()  [unwired: 2 in, 2 out]
            n414 = property on="sample" class="Slide (strict)"("DisabledEnum"=w431) -> ()  [unwired: 2 in, 2 out]
            n415 = property on="block" class="Slide (strict)"("DisabledEnum"=w431) -> ()  [unwired: 2 in, 2 out]
            n416 = case shown="False" w432 {
              tunnel: w431 -> [w443 _]
              frame False {
                n417 = property on="no.of samples (nos)" class="DigNum (strict)"("DisabledEnum"=w443) -> ()  [unwired: 2 in, 2 out]
              }
              frame True {
              }
            }
            n418 = property on="alloc mem" class="Bool (strict)"("DisabledEnum"=w431) -> ()  [unwired: 2 in, 2 out]
            n419 = call "contFFLoop.vi"("Numeric"=w434) -> ()  [unwired: 1 in]
            n420 = property on="Scan Trig Input Sel" class="CmbBox"() -> ("Value"=w423:string)  [unwired: 2 in, 2 out]
            n421 = property on="fast test\ncontinuous" class="Bool (strict)"("DisabledEnum"=w433) -> ()  [unwired: 2 in, 2 out]
            n422 = property on="fast test\ncontinuous" class="Bool (strict)"("Value"=w430) -> ()  [unwired: 2 in, 2 out]
            n423 = global read "Globals.vi" "mshut"() -> (w428:bool)
            n424 = case shown="\"Intern\"" w423 {
              tunnel: [TRUE FALSE] -> w422
              frame "Intern" {
              }
              frame Default {
              }
            }
            n425 = property on="is FFT" class="Bool (strict)"() -> ("Value"=w426:bool)  [unwired: 2 in, 2 out]
            n426 = Not(x=w428) -> (.not. x?=w427:bool)
            n427 = And(x=w426, y=w427) -> (x .and. y?=w425:bool)
            n428 = And(x=w425, y=w422) -> (x .and. y?=w424:bool)
            n429 = case shown="True" w424 {
              tunnel: [FALSE w439] -> w429
              frame False {
              }
              frame True {
                n430 = property on="FFT mode" class="CmbBox"() -> ("Value"=w440:string)  [unwired: 2 in, 2 out]
                n431 = case shown="\"Area\", \"Region of Interest\"" w440 {
                  tunnel: [FALSE w442] -> w439
                  frame Default {
                  }
                  frame "Area", "Region of Interest" {
                    n432 = property on="framewise\ncontinuous" class="Bool (strict)"() -> ("Value"=w442:bool)  [unwired: 2 in, 2 out]
                  }
                }
              }
            }
            n433 = property on="String" class="Str"("Blinking"=w429) -> ()  [unwired: 2 in, 2 out]
            n434 = property on="String" class="Str"("Visible"=w429) -> ()  [unwired: 2 in, 2 out]
          }
          event "fast test\ncontinuous": Value Change {
            # "2 because with 1 the old \ncont mode is set"
            # "setting continuos mode"
            n435 = event-data() -> ()  [unwired: 1 in, 6 out]
            n436 = case shown="True" "fast test\ncontinuous" {
              tunnel: [0 2] -> w452
              frame False {
                n437 = property on="no.of samples (nos)" class="DigNum (strict)"() -> ("Value"=w456:u32)  [unwired: 2 in, 2 out]
                n438 = property on="alloc mem" class="Bool (strict)"() -> ("Value"=w457:bool)  [unwired: 2 in, 2 out]
                n439 = property on="alloc mem" class="Bool (strict)"("Val(Sgnl)"=w457) -> ()  [unwired: 2 in, 2 out]
                n440 = property on="no.of samples (nos)" class="DigNum (strict)"("Val(Sgnl)"=w456) -> ()  [unwired: 2 in, 2 out]
              }
              frame True {
                w462 = u32 1
                # "Setup DMA"
                n441 = property on="FFT mode" class="CmbBox"() -> ("Value"=w460:string)  [unwired: 2 in, 2 out]
                n442 = property on="exposuretime[ms]" class="DigNum (strict)"() -> ("Value"=w461:dbl)  [unwired: 2 in, 2 out]
                n443 = case shown="Default" w460 {
                  tunnel: [w465 w467] -> w459
                  tunnel: w461 -> [_ w466]
                  frame "Area", "Region of Interest" {
                    n444 = global read "Globals.vi" "nos"() -> (w465:u32)
                  }
                  frame Default {
                    w472 = u32 2
                    n445 = Divide(x=u32 50, y=w466) -> (x/y=w469:dbl)
                    n446 = To Unsigned Long Integer(number=w469) -> (unsigned 32bit integer=w471:u32)
                    n447 = Less?(x=w471, y=w472) -> (x < y?=w470:bool)
                    n448 = case shown="False" w470 {
                      tunnel: w471 -> [w473 _]
                      tunnel: [w473 w474] -> w467
                      tunnel: w472 -> [_ w474]
                      frame False {
                      }
                      frame True {
                      }
                    }
                    n449 = property on="sample" class="Slide (strict)"("Value"=w467) -> ()  [unwired: 2 in, 2 out]
                    n450 = property on="no.of samples (nos)" class="DigNum (strict)"("Value"=w467) -> ()  [unwired: 2 in, 2 out]
                    n451 = global write "Globals.vi" "nos"(w467) -> ()
                  }
                }
                n452 = property on="block" class="Slide (strict)"("Value"=w462) -> ()  [unwired: 2 in, 2 out]
                n453 = global write "Globals.vi" "nob"(w462) -> ()
                n454 = property on="no.of blocks (nob)" class="DigNum (strict)"("Value"=w462) -> ()  [unwired: 2 in, 2 out]
                n455 = global read "Globals.vi" "board_sel"() -> (w464:u32)
                n456 = call "SetupDMA_thread.vi"("blocks"=w462, "nos"=w459, "Board_sel"=w464) -> ()  [unwired: 2 in]
              }
            }
            n457 = property on="is FFT" class="Bool (strict)"() -> ("Value"=w453:bool)  [unwired: 2 in, 2 out]
            n458 = property on="no.of blocks (nob)" class="DigNum (strict)"("DisabledEnum"=w452) -> ()  [unwired: 2 in, 2 out]
            n459 = property on="sample" class="Slide (strict)"("DisabledEnum"=w452) -> ()  [unwired: 2 in, 2 out]
            n460 = property on="block" class="Slide (strict)"("DisabledEnum"=w452) -> ()  [unwired: 2 in, 2 out]
            n461 = case shown="False" w453 {
              tunnel: w452 -> [w455 _]
              frame False {
                n462 = property on="no.of samples (nos)" class="DigNum (strict)"("DisabledEnum"=w455) -> ()  [unwired: 2 in, 2 out]
              }
              frame True {
              }
            }
            n463 = property on="alloc mem" class="Bool (strict)"("DisabledEnum"=w452) -> ()  [unwired: 2 in, 2 out]
          }
          event "alloc mem": Value Change {
            w477 = u32 10
            w481 = 0
            # "trigger dac update"
            # "cursor jumps to the left"
            # "Setup DMA"
            # "update params"
            n464 = event-data() -> ()  [unwired: 1 in, 6 out]
            n465 = property on="send all" class="Bool (strict)"() -> ("Value"=w483:bool)  [unwired: 2 in, 2 out]
            n466 = global read "Globals.vi" "board_sel"() -> (w487:u32)
            n467 = global read "Globals.vi" "nos"() -> (w486:u32)
            n468 = global read "Globals.vi" "nob"() -> (w485:u32)
            n469 = call "SetupDMA_thread.vi"("blocks"=w485, "nos"=w486, "Board_sel"=w487) -> ()  [unwired: 2 in]
            n470 = property on="send all" class="Bool (strict)"("Val(Sgnl)"=w483) -> ()  [unwired: 2 in, 2 out]
            n471 = property on="show greyscale viewer" class="Bool (strict)"("DisabledEnum"=0) -> ()  [unwired: 2 in, 2 out]
            n472 = property on="TRMS Pix" class="DigNum (strict)"("DisabledEnum"=w481) -> ()  [unwired: 2 in, 2 out]
            n473 = property on="start" class="Bool (strict)"("DisabledEnum"=w481) -> ()  [unwired: 2 in, 2 out]
            n474 = property on="sample" class="Slide (strict)"("DisabledEnum"=w481) -> ()  [unwired: 2 in, 2 out]
            n475 = property on="framewise\ncontinuous" class="Bool (strict)"("DisabledEnum"=w481) -> ()  [unwired: 2 in, 2 out]
            n476 = property on="block" class="Slide (strict)"("DisabledEnum"=w481) -> ()  [unwired: 2 in, 2 out]
            n477 = global read "Globals.vi" "nos"() -> (w475:u32)
            n478 = property on="exposuretime[ms]" class="DigNum (strict)"() -> ("Value"=w488:dbl)  [unwired: 2 in, 2 out]
            n479 = property on="DAT in 10ns" class="DigNum (strict)"() -> ("Value"=w484:u32)  [unwired: 2 in, 2 out]
            n480 = property on="block" class="Slide (strict)"("Value"=u32 1) -> ()  [unwired: 2 in, 2 out]
            n481 = Less?(x=w477, y=w475) -> (x < y?=w478:bool)
            n482 = property on="DAT in 10ns" class="DigNum (strict)"("Val(Sgnl)"=w484) -> ()  [unwired: 2 in, 2 out]
            n483 = case shown="False" w478 {
              tunnel: w477 -> [_ w490]
              tunnel: [w489 w490] -> w476
              tunnel: w475 -> [w489 _]
              frame False {
              }
              frame True {
              }
            }
            n484 = property on="exposuretime[ms]" class="DigNum (strict)"("Val(Sgnl)"=w488) -> ()  [unwired: 2 in, 2 out]
            n485 = property on="rep time" class="DigNum (strict)"() -> ("Value"=w479:dbl)  [unwired: 2 in, 2 out]
            n486 = property on="sample" class="Slide (strict)"("Value"=w476) -> ()  [unwired: 2 in, 2 out]
            n487 = property on="rep time" class="DigNum (strict)"("Val(Sgnl)"=w479) -> ()  [unwired: 2 in, 2 out]
          }
          event "show greyscale viewer": Value Change {
            n488 = event-data() -> ()  [unwired: 1 in, 6 out]
            n489 = case shown="True" "show greyscale viewer" {
              frame False {
                n490 = call "deinit2dViewer.vi"() -> ()  [unwired: 5 in]
              }
              frame True {
                n491 = flat-sequence {
                  frame #0 {
                    n492 = global read "Globals.vi" "board_sel"() -> (w492:u32)
                    n493 = global read "Globals.vi" "nos"() -> (w496:u32)
                    n494 = global read "Globals.vi" "PIXEL"() -> (w495:u32)
                    n495 = call "show2dViewer.vi"("nos"=w496, "pixel"=w495, "cam"=u16 0, "cur_nob"=u16 0, "drvno"=w492) -> ()
                  }
                  frame #1 {
                    n496 = property on="value black" class="DigNum (strict)"() -> ("Value"=w499:u32)  [unwired: 2 in, 2 out]
                    n497 = property on="value white" class="DigNum (strict)"() -> ("Value"=w498:u32)  [unwired: 2 in, 2 out]
                    n498 = property on="sample" class="Slide (strict)"() -> ("Value"=w497:u32)  [unwired: 2 in, 2 out]
                    n499 = property on="sample" class="Slide (strict)"("Val(Sgnl)"=w497) -> ()  [unwired: 2 in, 2 out]
                    n500 = call "setGamma.vi"("black"=w499, "white"=w498) -> ()  [unwired: 1 in]
                  }
                }
              }
            }
          }
          event "start": Mouse Down {
            # "start measurement"
            n501 = event-data() -> ()  [unwired: 1 in, 8 out]
            n502 = global read "Globals.vi" "mshut"() -> (w500:bool)
            n503 = property on="refresh" class="Bool (strict)"("Val(Sgnl)"="refresh") -> ()  [unwired: 2 in, 2 out]
            n504 = case shown="True" w500 {
              frame False {
                n505 = property on="startevent" class="Bool (strict)"() -> ("Value"=w504:bool)  [unwired: 2 in, 2 out]
                n506 = property on="startevent" class="Bool (strict)"("Val(Sgnl)"=w504) -> ()  [unwired: 2 in, 2 out]
              }
              frame True {
                # "limit for the shutter \nin ms"
                n507 = property on="rep time" class="DigNum (strict)"() -> ("Value"=w505:dbl)  [unwired: 2 in, 2 out]
                n508 = Less?(x=w505, y=20.0) -> (x < y?=w506:bool)
                n509 = case shown="False" w506 {
                  frame False {
                    n510 = property on="startevent" class="Bool (strict)"() -> ("Value"=w508:bool)  [unwired: 2 in, 2 out]
                    n511 = property on="startevent" class="Bool (strict)"("Val(Sgnl)"=w508) -> ()  [unwired: 2 in, 2 out]
                  }
                  frame True {
                    n512 = call "Display Message to User3"() -> ("no"=w509:bool)  [unwired: 10 in, 1 out]
                    n513 = case shown="False" w509 {
                      frame False {
                        n514 = property on="startevent" class="Bool (strict)"("Val(Sgnl)"="startevent") -> ()  [unwired: 2 in, 2 out]
                      }
                      frame True {
                      }
                    }
                  }
                }
              }
            }
            n515 = case shown="True" FALSE {
              frame False {
              }
              frame True {
                w511 = u8 5 items=["S0Addr_CtrlA"=4, "S0Addr_CtrlB"=5, "S0Addr_CtrlC"=6, "S0Addr_XCKLL"=8, "S0Addr_XCKLH"=9, "S0Addr_XCKHL"=10, "S0Addr_XCKMSB"=11, "S0Addr_XCKCNTLL"=12, "S0Addr_XCKCNTLH"=13, "S0Addr_XCKCNTHL"=14, "S0Addr_XCKCNTMSB"=15, "S0Addr_PIXREGlow"=16, "S0Addr_PIXREGhigh"=17, "S0Addr_FREQREG"=18, "S0Addr_FF_FLAGS"=19, "S0Addr_FIFOCNT"=20, "S0Addr_VCLKCTRL"=24, "S0Addr_EBST"=28, "S0Addr_DAT"=32, "S0Addr_EC"=36, "S0Addr_TOR"=40, "S0Addr_ARREG"=44, "S0Addr_GIOREG"=48, "S0Addr_DELAYEC"=52, "S0Addr_IRQREG"=56, "S0Addr_PCI"=60]
                # "CtrlB register @ 0x05"
                n516 = call "WriteB.vi"("val"=u8 33, "offset"=w511) -> ()
              }
            }
            n517 = property on="Offset" class="Bool (strict)"() -> ("Value"=w503:bool)  [unwired: 2 in, 2 out]
            n518 = case shown="True" w503 {
              frame False {
                n519 = global write "Globals.vi" "board_sel_offset"(u32 1) -> ()
              }
              frame True {
                n520 = global write "Globals.vi" "board_sel_offset"(u32 2) -> ()
              }
            }
          }
          event "startevent": Value Change {
            # "block trigger input\n0: internal -> next block is started immediately \n1: external -> I- input\n2: external -> S1- input\n3: external -> S2- input\n4: external -> S1&S2- input"
            # "only 1st PCI board is used for ext. trig."
            # "ext. scan trig\n0: internal: timer\n1: external"
            # "block trigger\n0: internal -> next block is started immediately \n1: external -> all blocks on one trigger\n2: external -> one block per trigger"
            n521 = event-data() -> ()  [unwired: 1 in, 6 out]
            n522 = global read "Globals.vi" "exp time"() -> (w525:dbl)
            n523 = property on="BlockSyncStart" class="CmbBox"() -> ("Value"=w518:string)  [unwired: 2 in, 2 out]
            n524 = property on="Scan Trig Input Sel" class="CmbBox"() -> ("Value"=w520:string)  [unwired: 2 in, 2 out]
            n525 = property on="Scan Trig Input Sel" class="CmbBox"() -> ("Value"=w521:string)  [unwired: 2 in, 2 out]
            n526 = case shown="Default" w518 {
              tunnel: [TRUE FALSE] -> w517
              frame Default {
              }
              frame "Intern" {
              }
            }
            n527 = case shown="\"Intern\"" w520 {
              tunnel: [FALSE TRUE] -> w519
              frame Default {
              }
              frame "Intern" {
              }
            }
            n528 = Multiply(x=1000.0, y=w525) -> (x*y=w523:dbl)
            n529 = To Unsigned Long Integer(number=w523) -> (unsigned 32bit integer=w527:u32)
            n530 = case shown="Default" w521 {
              tunnel: [u8 1 u8 0] -> w526
              frame Default {
              }
              frame "Intern" {
              }
            }
            n531 = global read "Globals.vi" "board_sel"() -> (w528:u32)
            n532 = And(x=w517, y=w519) -> (x .and. y?=w522:bool)
            n533 = case shown="True" w522 {
              tunnel: [u8 0 u8 2] -> _
              frame False {
              }
              frame True {
              }
            }
            n534 = global read "Globals.vi" "block_ch"() -> (w515:u8)
            n535 = call "ReadFFLoop_thread.vi"("board_sel"=w528, "exptus"=w527, "ExtTrig"=w526, "btrig_ch"=w515, "blocktrigger"=u8 2) -> ()
          }
          event "start": Mouse Up {
            w537 = 0
            # "refresh trms and signalgraph if measurtime is too short for the Measure On LED (<100ms / Timeout)"
            n536 = event-data() -> ()  [unwired: 1 in, 8 out]
            n537 = property on="DAC 3/ 1" class="DigNum (strict)"("DisabledEnum"=w537) -> ()  [unwired: 2 in, 2 out]
            n538 = property on="DAC 1/ 1" class="DigNum (strict)"("DisabledEnum"=w537) -> ()  [unwired: 2 in, 2 out]
            n539 = property on="DAC 2/ 1" class="DigNum (strict)"("DisabledEnum"=w537) -> ()  [unwired: 2 in, 2 out]
            n540 = property on="DAC 4/ 1" class="DigNum (strict)"("DisabledEnum"=w537) -> ()  [unwired: 2 in, 2 out]
            n541 = property on="TRMS Pix" class="DigNum (strict)"() -> ("Value"=w540:u32)  [unwired: 2 in, 2 out]
            n542 = property on="Pixel for Graph" class="Slide (strict)"() -> ("Value"=w538:u32)  [unwired: 2 in, 2 out]
            n543 = property on="sample" class="Slide (strict)"() -> ("Value"=w539:u32)  [unwired: 2 in, 2 out]
            n544 = property on="DAC 6/ 1" class="DigNum (strict)"("DisabledEnum"=w537) -> ()  [unwired: 2 in, 2 out]
            n545 = property on="DAC 7/ 1" class="DigNum (strict)"("DisabledEnum"=w537) -> ()  [unwired: 2 in, 2 out]
            n546 = property on="DAC 5/ 1" class="DigNum (strict)"("DisabledEnum"=w537) -> ()  [unwired: 2 in, 2 out]
            n547 = property on="DAC 8/ 1" class="DigNum (strict)"("DisabledEnum"=w537) -> ()  [unwired: 2 in, 2 out]
            n548 = property on="TRMS Pix" class="DigNum (strict)"("Val(Sgnl)"=w540) -> ()  [unwired: 2 in, 2 out]
            n549 = property on="Pixel for Graph" class="Slide (strict)"("Val(Sgnl)"=w538) -> ()  [unwired: 2 in, 2 out]
            n550 = property on="sample" class="Slide (strict)"("Val(Sgnl)"=w539) -> ()  [unwired: 2 in, 2 out]
            n551 = property on="Offset" class="Bool (strict)"("DisabledEnum"=w537) -> ()  [unwired: 2 in, 2 out]
            n552 = property on="send all" class="Bool (strict)"("DisabledEnum"=w537) -> ()  [unwired: 2 in, 2 out]
          }
          event "sample", "block": Value Change {
            n553 = event-data() -> ()  [unwired: 1 in, 6 out]
            n554 = stacked-sequence {
              frame #0 {
                w564 = u32 1
                # "when selecting a value\nbigger than possible\nnos or nob, a dummy \nvalue \"1\" is chosen\n\nTODO:\ninsert error handling\nwith lower values than 1"
                # "display"
                n555 = global read "Globals.vi" "board_sel"() -> (w552:u32)
                n556 = global read "Globals.vi" "nos"() -> (w563:u32)
                n557 = global read "Globals.vi" "nob"() -> (w558:u32)
                n558 = global read "Globals.vi" "boards"() -> (w554:u32)
                n559 = Greater Or Equal?(x=w563, y="sample") -> (x >= y?=w556:bool)
                n560 = Greater Or Equal?(x=w558, y="block") -> (x >= y?=w555:bool)
                n561 = case shown="True" w556 {
                  tunnel: [u32 1 w640] -> w562
                  tunnel: "sample" -> [_ w640]
                  frame False {
                    n562 = call "Display Message to User2"() -> ()  [unwired: 10 in, 2 out]
                  }
                  frame True {
                  }
                }
                n563 = case shown="1, Default" w554 {
                  tunnel: [u32 1 w576] -> w553
                  tunnel: w552 -> [_ w576]
                  frame 1, Default {
                  }
                  frame 2 {
                  }
                }
                n564 = case shown="False" w555 {
                  tunnel: [u32 1 w638] -> w560
                  tunnel: "block" -> [_ w638]
                  frame False {
                    n565 = call "Display Message to User"() -> ()  [unwired: 10 in, 2 out]
                  }
                  frame True {
                  }
                }
                n566 = Subtract(x=w562, y=w564) -> (x-y=w544:u32)
                n567 = Subtract(x=w560, y=w564) -> (x-y=w542:u32)
                n568 = case shown="2, 3" w553 {
                  tunnel: w544 -> [_ w647]
                  tunnel: w542 -> [_ w645]
                  frame 1, Default {
                  }
                  frame 2, 3 {
                    n569 = global read "Globals.vi" "PIXEL"() -> (w643:u32)
                    n570 = To Long Integer(number=w643) -> (32bit integer=w644:i32)
                    n571 = Initialize Array(u16 100, w644) -> (w649:u16[])
                    n572 = call "ReturnFrame.vi"("curr_cam"=u16 0, "length"=w643, "Data Values In"=w649, "curr_nob"=w645, "curr_nos"=w647, "Drv"=u32 2) -> ("Data Values Out"=→"Signal Board 2 / Cam1":u16[])
                  }
                }
                n573 = global read "Globals.vi" "board_sel"() -> (w551:u32)
                n574 = global read "Globals.vi" "CAMCNT"() -> (w557:u32)
                n575 = case shown="1, 3" w551 {
                  tunnel: w542 -> [_ w569]
                  tunnel: w544 -> [_ w568]
                  frame 2, Default {
                  }
                  frame 1, 3 {
                    n576 = global read "Globals.vi" "PIXEL"() -> (w566:u32)
                    n577 = To Long Integer(number=w566) -> (32bit integer=w574:i32)
                    n578 = Initialize Array(u16 100, w574) -> (w570:u16[])
                    n579 = global read "Globals.vi" "PIXEL"() -> (w565:u32)
                    n580 = call "ReturnFrame.vi"("curr_cam"=u16 0, "length"=w565, "Data Values In"=w570, "curr_nob"=w569, "curr_nos"=w568, "Drv"=u32 1) -> ("Data Values Out"=→"Signal Board 1 / Cam1":u16[])
                  }
                }
                n581 = case shown="1, Default" w557 {
                  tunnel: w542 -> [_ w590 w598 w619]
                  tunnel: w544 -> [_ w581 w594 w614]
                  tunnel: [w577 w587 w601 w626] -> w550
                  tunnel: [w577 w583 w600 w625] -> w549
                  tunnel: [w577 w583 w599 w618] -> w548
                  frame 1, Default {
                    n582 = To Long Integer(number=u16 1088) -> (32bit integer=w578:i32)
                    n583 = Initialize Array(u16 0, w578) -> (w577:u16[])
                  }
                  frame 2 {
                    n584 = global read "Globals.vi" "PIXEL"() -> (w588:u32)
                    n585 = To Long Integer(number=u16 1088) -> (32bit integer=w584:i32)
                    n586 = To Long Integer(number=w588) -> (32bit integer=w589:i32)
                    n587 = Initialize Array(u16 0, w584) -> (w583:u16[])
                    n588 = Initialize Array(u16 100, w589) -> (w591:u16[])
                    n589 = call "ReturnFrame.vi"("curr_cam"=u16 1, "length"=w588, "Data Values In"=w591, "curr_nob"=w590, "curr_nos"=w581, "Drv"=u32 1) -> ("Data Values Out"=w587:u16[])
                  }
                  frame 3 {
                    n590 = global read "Globals.vi" "PIXEL"() -> (w596:u32)
                    n591 = global read "Globals.vi" "PIXEL"() -> (w609:u32)
                    n592 = To Long Integer(number=u16 1088) -> (32bit integer=w606:i32)
                    n593 = To Long Integer(number=w596) -> (32bit integer=w602:i32)
                    n594 = To Long Integer(number=w609) -> (32bit integer=w610:i32)
                    n595 = Initialize Array(u16 0, w606) -> (w599:u16[])
                    n596 = Initialize Array(u16 100, w602) -> (w603:u16[])
                    n597 = Initialize Array(u16 100, w610) -> (w611:u16[])
                    n598 = call "ReturnFrame.vi"("curr_cam"=u16 2, "length"=w596, "Data Values In"=w603, "curr_nob"=w598, "curr_nos"=w594, "Drv"=u32 1) -> ("Data Values Out"=w600:u16[])
                    n599 = call "ReturnFrame.vi"("curr_cam"=u16 1, "length"=w609, "Data Values In"=w611, "curr_nob"=w598, "curr_nos"=w594, "Drv"=u32 1) -> ("Data Values Out"=w601:u16[])
                  }
                  frame 4 {
                    n600 = global read "Globals.vi" "PIXEL"() -> (w620:u32)
                    n601 = global read "Globals.vi" "PIXEL"() -> (w627:u32)
                    n602 = global read "Globals.vi" "PIXEL"() -> (w632:u32)
                    n603 = To Long Integer(number=w620) -> (32bit integer=w621:i32)
                    n604 = To Long Integer(number=w627) -> (32bit integer=w628:i32)
                    n605 = To Long Integer(number=w632) -> (32bit integer=w633:i32)
                    n606 = Initialize Array(u16 100, w621) -> (w622:u16[])
                    n607 = Initialize Array(u16 100, w628) -> (w629:u16[])
                    n608 = Initialize Array(u16 100, w633) -> (w634:u16[])
                    n609 = call "ReturnFrame.vi"("curr_cam"=u16 3, "length"=w620, "Data Values In"=w622, "curr_nob"=w619, "curr_nos"=w614, "Drv"=u32 1) -> ("Data Values Out"=w618:u16[])
                    n610 = call "ReturnFrame.vi"("curr_cam"=u16 2, "length"=w627, "Data Values In"=w629, "curr_nob"=w619, "curr_nos"=w614, "Drv"=u32 1) -> ("Data Values Out"=w625:u16[])
                    n611 = call "ReturnFrame.vi"("curr_cam"=u16 1, "length"=w632, "Data Values In"=w634, "curr_nob"=w619, "curr_nos"=w614, "Drv"=u32 1) -> ("Data Values Out"=w626:u16[])
                  }
                }
                "Signal Cam 2" <- w550
                "Signal Cam 3" <- w549
                "Signal Cam 4" <- w548
                n612 = global read "Globals.vi" "board_sel"() -> (w547:u32)
                n613 = To Unsigned Word Integer(number=w542) -> (unsigned 16bit integer=w543:u16)
                n614 = global read "Globals.vi" "PIXEL"() -> (w546:u32)
                n615 = global read "Globals.vi" "nos"() -> (w545:u32)
                n616 = call "update2dViewer.vi"("nos"=w545, "pixel"=w546, "cam"=u16 0, "cur_nob"=w543, "drvno"=w547) -> ()
              }
              frame #1 {
                w651 = 3
                # "3 channel per tdc"
                n617 = property on="Signal Board 1 / Cam1" class="WFGraph (strict)"() -> ("Value"=w658:u16[])  [unwired: 2 in, 2 out]
                n618 = Index Array(array=w658, index=7) -> (element=w659:u16)
                n619 = Index Array(array=w658, index=6) -> (element=w661:u16)
                n620 = And(x=w659, y=u16 65535) -> (x .and. y?=w650:u16)
                n621 = And(x=w661, y=u16 65535) -> (x .and. y?=w652:u16)
                n622 = Divide(x=w652, y=w651) -> (x/y=w653:dbl)
                n623 = global read "Globals.vi" "GPX Offset"() -> (w657:u32)
                n624 = Divide(x=w650, y=w651) -> (x/y=w656:dbl)
                n625 = Subtract(x=w653, y=w657) -> (x-y=→"TDC 1":dbl)
                n626 = Subtract(x=w656, y=w657) -> (x-y=→"TDC 2":dbl)
              }
            }
          }
          event "Pixel for Graph": Value Change {
            n627 = event-data() -> ()  [unwired: 1 in, 6 out]
            n628 = global read "Globals.vi" "nob"() -> (w666:u32)
            n629 = for {
              N: w666 -> [_]
              tunnel: [w667] -> w665 mode=indexing
              i -> [w668]
              n630 = global read "Globals.vi" "nos"() -> (w669:u32)
              n631 = for {
                N: w669 -> [_]
                tunnel: w668 -> [w674]
                tunnel: [w672] -> w667 mode=indexing
                i -> [w675]
                n632 = global read "Globals.vi" "PIXEL"() -> (w676:u32)
                n633 = To Long Integer(number=w676) -> (32bit integer=w677:i32)
                n634 = Initialize Array(u16 100, w677) -> (w680:u16[])
                n635 = call "ReturnFrame.vi"("curr_cam"=u16 0, "length"=w676, "Data Values In"=w680, "curr_nob"=w674, "curr_nos"=w675, "Drv"=u32 1) -> ("Data Values Out"=w673:u16[])
                n636 = Index Array(array=w673, index="Pixel for Graph") -> (element=w672:u16)
              }
            }
            "One Pixel Graph" <- w665
          }
          event "About S0": Mouse Down {
            n637 = event-data() -> ()  [unwired: 1 in, 8 out]
            n638 = call "aboutS0.vi"() -> ()  [unwired: 1 in]
          }
          event "DAT in 10ns": Value Change {
            # "bit31 must be set for enabling DAT(add 0x80000000) to REG 0x20"
            # "is only valid for external trigger!"
            # "this examples shows how to set the DAT (delay after trigger)"
            n639 = event-data() -> ()  [unwired: 1 in, 6 out]
            n640 = Equal To 0?(x="DAT in 10ns") -> (x = 0?=w682:bool)
            n641 = case shown="False" w682 {
              tunnel: "DAT in 10ns" -> [w686 _]
              frame False {
                w683 = u8 32 items=["S0Addr_CtrlA"=4, "S0Addr_CtrlB"=5, "S0Addr_CtrlC"=6, "S0Addr_XCKLL"=8, "S0Addr_XCKLH"=9, "S0Addr_XCKHL"=10, "S0Addr_XCKMSB"=11, "S0Addr_XCKCNTLL"=12, "S0Addr_XCKCNTLH"=13, "S0Addr_XCKCNTHL"=14, "S0Addr_XCKCNTMSB"=15, "S0Addr_PIXREGlow"=16, "S0Addr_PIXREGhigh"=17, "S0Addr_FREQREG"=18, "S0Addr_FF_FLAGS"=19, "S0Addr_FIFOCNT"=20, "S0Addr_VCLKCTRL"=24, "S0Addr_EBST"=28, "S0Addr_DAT"=32, "S0Addr_EC"=36, "S0Addr_TOR"=40, "S0Addr_ARREG"=44, "S0Addr_GIOREG"=48, "S0Addr_DELAYEC"=52, "S0Addr_IRQREG"=56, "S0Addr_PCI"=60]
                n642 = global read "Globals.vi" "board_sel"() -> (w685:u32)
                n643 = Add(x=u32 2147483648, y=w686) -> (x+y=w684:u32)
                n644 = call "WriteL_thread.vi"("val"=w684, "board_sel"=w685, "offset"=w683) -> ()
              }
              frame True {
                w688 = u8 32 items=["S0Addr_CtrlA"=4, "S0Addr_CtrlB"=5, "S0Addr_CtrlC"=6, "S0Addr_XCKLL"=8, "S0Addr_XCKLH"=9, "S0Addr_XCKHL"=10, "S0Addr_XCKMSB"=11, "S0Addr_XCKCNTLL"=12, "S0Addr_XCKCNTLH"=13, "S0Addr_XCKCNTHL"=14, "S0Addr_XCKCNTMSB"=15, "S0Addr_PIXREGlow"=16, "S0Addr_PIXREGhigh"=17, "S0Addr_FREQREG"=18, "S0Addr_FF_FLAGS"=19, "S0Addr_FIFOCNT"=20, "S0Addr_VCLKCTRL"=24, "S0Addr_EBST"=28, "S0Addr_DAT"=32, "S0Addr_EC"=36, "S0Addr_TOR"=40, "S0Addr_ARREG"=44, "S0Addr_GIOREG"=48, "S0Addr_DELAYEC"=52, "S0Addr_IRQREG"=56, "S0Addr_PCI"=60]
                n645 = global read "Globals.vi" "board_sel"() -> (w690:u32)
                n646 = call "WriteL_thread.vi"("val"=u32 0, "board_sel"=w690, "offset"=w688) -> ()
              }
            }
          }
          event "no.of samples (nos)", "no.of blocks (nob)", "exposuretime[ms]", "rep time": Value Change {
            # "set EC"
            # "calculation of MB RAM an SEC and setting scale max"
            n647 = event-data() -> ()  [unwired: 1 in, 7 out]
            n648 = global read "Globals.vi" "mshut"() -> (w701:bool)
            n649 = global read "Globals.vi" "nob"() -> (w703:u32)
            n650 = global read "Globals.vi" "nos"() -> (w705:u32)
            n651 = global write "Globals.vi" "nos"("no.of samples (nos)") -> ()
            n652 = To Double Precision Float(number=w705) -> (double precision float=w704:dbl)
            n653 = To Double Precision Float(number=w703) -> (double precision float=w702:dbl)
            n654 = global write "Globals.vi" "nob"("no.of blocks (nob)") -> ()
            n655 = case shown="True" w701 {
              tunnel: [w713 w714] -> w696
              tunnel: "exposuretime[ms]" -> [w713 _]
              tunnel: "rep time" -> [_ w714]
              frame False {
              }
              frame True {
              }
            }
            n656 = property on="sample" class="Slide (strict)"("Scale.Maximum"=w704) -> ()  [unwired: 2 in, 2 out]
            n657 = property on="block" class="Slide (strict)"("Scale.Maximum"=w702) -> ()  [unwired: 2 in, 2 out]
            n658 = global read "Globals.vi" "nob"() -> (w693:u32)
            n659 = global write "Globals.vi" "exp time"(w696) -> ()
            n660 = global read "Globals.vi" "nos"() -> (w694:u32)
            n661 = global read "Globals.vi" "nob"() -> (w697:u32)
            n662 = global read "Globals.vi" "nos"() -> (w698:u32)
            n663 = call "CalcRamUsage.vi"("nob"=w693, "nos"=w694) -> ("ramUsage"=→"MB RAM":dbl)
            n664 = call "CalcMeasureTimeInSeconds.vi"("exposure_time_in_ms"=w696, "nob"=w697, "nos"=w698) -> ("measureTimeInSeconds"=→"SEC":dbl)
            n665 = global read "Globals.vi" "mshut"() -> (w691:bool)
            n666 = case shown="True" w691 {
              frame False {
                n667 = global read "Globals.vi" "board_sel"() -> (w708:u32)
                n668 = call "ResetEC.vi"("board_sel"=w708) -> ()  [unwired: 2 in]
              }
              frame True {
                n669 = property on="exposuretime[ms]" class="DigNum (strict)"() -> ("Value"=w709:dbl)  [unwired: 2 in, 2 out]
                n670 = global read "Globals.vi" "board_sel"() -> (w712:u32)
                n671 = Multiply(x=w709, y=100000.0) -> (x*y=w711:dbl)
                n672 = call "SetEC.vi"("ecin100ns"=w711, "board_sel"=w712) -> ()  [unwired: 1 in]
              }
            }
          }
          event "stop all": Value Change {
            # "exit"
            n673 = event-data() -> ()  [unwired: 1 in, 6 out]
            n674 = stacked-sequence {
              tunnel: [_ _ TRUE] -> w715
              frame #0 {
                n675 = property on="show greyscale viewer" class="Bool (strict)"("Value"=FALSE) -> ()  [unwired: 2 in, 2 out]
                n676 = call "deinit2dViewer.vi"() -> ()  [unwired: 5 in]
              }
              frame #1 {
                n677 = call "FFStop.vi"() -> ()  [unwired: 1 in]
              }
              frame #2 {
                # "do not omit, or next call of driver will go wrong."
                n678 = global read "Globals.vi" "board_sel"() -> (w717:u32)
                n679 = call "Exit.vi"("board_sel"=w717) -> ()  [unwired: 1 in]
              }
            }
          }
          event "TRMS Pix": Value Change {
            w723 = u32 300
            # "CHA"
            n680 = event-data() -> ()  [unwired: 1 in, 6 out]
            n681 = global read "Globals.vi" "CAMCNT"() -> (w721:u32)
            n682 = global read "Globals.vi" "nos"() -> (w729:u32)
            n683 = Greater?(x=w729, y=w723) -> (0:w731:bool)
            n684 = Greater?(x=w721, y=u32 1) -> (0:w719:bool)
            n685 = case shown="True" w731 {
              tunnel: [w746 w747] -> w730
              tunnel: w723 -> [_ w747]
              tunnel: w729 -> [w746 _]
              frame False {
              }
              frame True {
              }
            }
            n686 = case shown="True" w719 {
              tunnel: w723 -> [_ w734]
              tunnel: "TRMS Pix" -> [_ w733]
              frame False {
              }
              frame True {
                # "CHB"
                n687 = global read "Globals.vi" "nos"() -> (w740:u32)
                n688 = Greater?(x=w740, y=w734) -> (0:w742:bool)
                n689 = case shown="True" w742 {
                  tunnel: [w744 w745] -> w741
                  tunnel: w734 -> [_ w745]
                  tunnel: w740 -> [w744 _]
                  frame False {
                  }
                  frame True {
                  }
                }
                n690 = global read "Globals.vi" "board_sel"() -> (w743:u32)
                n691 = call "CalcTrms.vi"("TRMSpix"=w733, "scans"=w741, "CAMpos"=u16 1, "board_sel"=w743) -> ("TRMS 2"=→"tRMS 3":dbl, "mean 2"=→"mean 3":dbl, "TRMS 1"=→"tRMSB":dbl, "mean 1"=→"meanB":dbl)
              }
            }
            n692 = global read "Globals.vi" "board_sel"() -> (w732:u32)
            n693 = call "CalcTrms.vi"("TRMSpix"="TRMS Pix", "scans"=w730, "CAMpos"=0, "board_sel"=w732) -> ("TRMS 2"=→"tRMS 2":dbl, "mean 2"=→"mean 2":dbl, "TRMS 1"=→"tRMSA":dbl, "mean 1"=→"meanA":dbl)
          }
          event "ADC mode", "custom patt: 14bits pattern hex (14bit)": Value Change {
            n694 = event-data() -> ()  [unwired: 1 in, 6 out]
            n695 = case shown="\"2\"" "ADC mode" {
              tunnel: [w754 w755 w756] -> w750
              frame "1" {
                w754 = u8 2  # adc mode
                # "Custom Pattern"
              }
              frame "2" {
                w755 = u8 1  # adc mode
                # "Ramp"
              }
              frame "3" {
                w756 = u8 0  # adc mode
                # "Normal Mode"
              }
            }
            n696 = global read "Globals.vi" "cam gain"() -> (w753:u32)
            n697 = global read "Globals.vi" "board_sel"() -> (w751:u32)
            n698 = To Unsigned Byte Integer(number=w753) -> (unsigned 8bit integer=w748:u8)
            n699 = call "InitCam3030.vi"("gain_high"=w748, "custom_pattern"="custom patt: 14bits pattern hex (14bit)", "adc_mode"=w750, "drvno"=w751) -> ()  [unwired: 1 in]
            "pattern dec" <- "custom patt: 14bits pattern hex (14bit)"
          }
          event "Offset": Value Change {
            n700 = event-data() -> ()  [unwired: 1 in, 6 out]
            n701 = flat-sequence {
              frame #0 {
                n702 = global read "Globals.vi" "board_sel"() -> (w757:u32)
                n703 = case shown="1" w757 {
                  frame 2 {
                    n704 = property on="Offset" class="Bool (strict)"("Value"=TRUE) -> ()  [unwired: 2 in, 2 out]
                  }
                  frame 3, Default {
                  }
                  frame 1 {
                    n705 = property on="Offset" class="Bool (strict)"("Value"=FALSE) -> ()  [unwired: 2 in, 2 out]
                  }
                }
              }
              frame #1 {
                n706 = case shown="False" "Offset" {
                  tunnel: [FALSE TRUE] -> w761
                  tunnel: [TRUE FALSE] -> w762
                  frame False {
                    n707 = global write "Globals.vi" "board_sel_offset"(u32 1) -> ()
                  }
                  frame True {
                    n708 = global write "Globals.vi" "board_sel_offset"(u32 2) -> ()
                  }
                }
                n709 = global read "Globals.vi" "use DAC"() -> (w760:bool)
                n710 = And(x=w761, y=w760) -> ()  [unwired: 1 out]
                n711 = And(x=w760, y=w762) -> (x .and. y?=w763:bool)
                n712 = property on="DAC 4/ 1" class="DigNum (strict)"("Visible"=w763) -> ()  [unwired: 2 in, 2 out]
                n713 = property on="DAC 2/ 1" class="DigNum (strict)"("Visible"=w763) -> ()  [unwired: 2 in, 2 out]
                n714 = property on="DAC 3/ 1" class="DigNum (strict)"("Visible"=w763) -> ()  [unwired: 2 in, 2 out]
                n715 = property on="DAC 1/ 1" class="DigNum (strict)"("Visible"=w763) -> ()  [unwired: 2 in, 2 out]
                n716 = property on="DAC 5/ 1" class="DigNum (strict)"("Visible"=w763) -> ()  [unwired: 2 in, 2 out]
                n717 = property on="DAC 7/ 1" class="DigNum (strict)"("Visible"=w763) -> ()  [unwired: 2 in, 2 out]
                n718 = property on="DAC 8/ 1" class="DigNum (strict)"("Visible"=w763) -> ()  [unwired: 2 in, 2 out]
                n719 = property on="DAC 6/ 1" class="DigNum (strict)"("Visible"=w763) -> ()  [unwired: 2 in, 2 out]
              }
            }
          }
          event "DAC 2/ 1", "DAC 7/ 1", "DAC 3/ 1", "DAC 8/ 1", "DAC 4/ 1", "DAC 5/ 1", "DAC 1/ 1", "DAC 6/ 1": Value Change {
            w772 = u8 6  # channel
            w775 = u8 3  # channel
            w778 = u8 7  # channel
            w781 = u8 5  # channel
            w784 = u8 1  # channel
            w787 = u8 4  # channel
            w790 = u8 2  # channel
            w793 = u8 0  # channel
            # "CHG"
            # "CHD"
            # "CHH"
            # "CHF"
            # "CHB"
            # "CHE"
            # "CHC"
            # "CHA"
            n720 = event-data() -> ()  [unwired: 1 in, 6 out]
            n721 = global read "Globals.vi" "board_sel"() -> (w794:u32)
            n722 = global read "Globals.vi" "board_sel"() -> (w785:u32)
            n723 = global read "Globals.vi" "board_sel"() -> (w791:u32)
            n724 = global read "Globals.vi" "board_sel"() -> (w776:u32)
            n725 = call "DAC_setOutput.vi"("board_sel"=w794, "output"="DAC 4/ 1", "channel"=w793) -> ()
            n726 = call "DAC_setOutput.vi"("board_sel"=w785, "output"="DAC 5/ 1", "channel"=w784) -> ()
            n727 = call "DAC_setOutput.vi"("board_sel"=w791, "output"="DAC 1/ 1", "channel"=w790) -> ()
            n728 = call "DAC_setOutput.vi"("board_sel"=w776, "output"="DAC 6/ 1", "channel"=w775) -> ()
            n729 = global read "Globals.vi" "board_sel"() -> (w779:u32)
            n730 = global read "Globals.vi" "board_sel"() -> (w773:u32)
            n731 = global read "Globals.vi" "board_sel"() -> (w782:u32)
            n732 = global read "Globals.vi" "board_sel"() -> (w788:u32)
            n733 = call "DAC_setOutput.vi"("board_sel"=w779, "output"="DAC 8/ 1", "channel"=w778) -> ()
            n734 = call "DAC_setOutput.vi"("board_sel"=w773, "output"="DAC 3/ 1", "channel"=w772) -> ()
            n735 = call "DAC_setOutput.vi"("board_sel"=w782, "output"="DAC 7/ 1", "channel"=w781) -> ()
            n736 = call "DAC_setOutput.vi"("board_sel"=w788, "output"="DAC 2/ 1", "channel"=w787) -> ()
          }
          event "send all": Value Change {
            n737 = event-data() -> ()  [unwired: 1 in, 6 out]
            n738 = property on="DAC 4/ 1" class="DigNum (strict)"() -> ("Value"=w795:u16)  [unwired: 2 in, 2 out]
            n739 = property on="DAC 4/ 1" class="DigNum (strict)"("Val(Sgnl)"=w795) -> ()  [unwired: 2 in, 2 out]
          }
          event "camera gain": Value Change {
            # "CamControl Reg:\ngain bit CC0\nLED off bit CC1\nData = 00h: LED on, gain low\nData = 01h: LED on, gain high\nData = 10h: LED off, gain low\nData = 11h: LED off, gain high"
            # "register address channel select"
            n740 = event-data() -> ()  [unwired: 1 in, 6 out]
            n741 = property on="camera gain" class="Bool (strict)"() -> ("Value"=w797:bool)  [unwired: 2 in, 2 out]
            n742 = global read "Globals.vi" "maddr of CAM"() -> (w799:u8)
            n743 = global read "Globals.vi" "board_sel"() -> (w796:u32)
            n744 = case shown="True" w797 {
              tunnel: [w801 w802] -> w798
              frame False {
                w801 = u16 0  # data (hex)
              }
              frame True {
                w802 = u16 1  # data (hex)
              }
            }
            n745 = call "SendFLCam.vi"("adadr"=u8 0, "data"=w798, "madr"=w799, "board_sel"=w796) -> ()
          }
          event "value white", "value black": Value Change {
            n746 = event-data() -> ()  [unwired: 1 in, 6 out]
            n747 = property on="sample" class="Slide (strict)"() -> ("Value"=w803:u32)  [unwired: 2 in, 2 out]
            n748 = property on="sample" class="Slide (strict)"("Val(Sgnl)"=w803) -> ()  [unwired: 2 in, 2 out]
            n749 = call "setGamma.vi"("black"="value black", "white"="value white") -> ()  [unwired: 1 in]
          }
          event "shutter open": Value Change {
            n750 = event-data() -> ("NewVal"=w806:bool)  [unwired: 1 in, 5 out]
            n751 = case shown="False" w806 {
              frame False {
                # "Close Shutter"
                n752 = global read "Globals.vi" "board_sel"() -> (w807:u32)
                n753 = call "closeshutter.vi"("board_sel"=w807) -> ()  [unwired: 1 in]
              }
              frame True {
                # "OpenS hutter"
                n754 = global read "Globals.vi" "board_sel"() -> (w808:u32)
                n755 = call "OpenShutter.vi"("board_sel"=w808) -> ()  [unwired: 1 in]
              }
            }
          }
        }
      }
    }
  }
